vi "STED Control V15.vi"() -> ()   [LabVIEW 2014]
uses:
  Controls/Button 2.ctl
  Type Defs/Image Acquisition Parameters.ctl
  Laser Controls.ctl
  Detectors.ctl
  Type Defs/P541.ctl
  Type Defs/M227.ctl
  Type Defs/P612.ctl
  Type Defs/M686.ctl
  Type Defs/P841.ctl
  Type Defs/ASI.ctl
  Type Defs/N664_V2.ctl
  Type Defs/STED Graph Controls.ctl
  Type Defs/Display Controls.ctl
  Type Defs/Z comp.ctl
  FPGA-7842R-Reference.ctl
  Manual Controls V2.ctl
  Scan Parameters.ctl
  <vilib>/Utility/miscctls.llb/LVPositionTypeDef.ctl
  Controls/StageStates.ctl
  DM_Dual_V2/Controls/Standard Action.ctl
  Focus Lock/Controls/Counter Action.ctl
  Focus Lock/Controls/Standard Action for Focus Lock.ctl
  <vilib>/Utility/miscctls.llb/LVRectTypeDef.ctl
  <vilib>/event_ctls.llb/lveventtype.ctl
  <vilib>/Utility/file.llb/Read From Spreadsheet File (DBL).vi
  <vilib>/FPGAPlugInAG/PCIe-7841R/niLvFpga_Open_PCIe-7841R.vi
  <vilib>/FPGAPlugInAG/PCIe-7841R/niLvFpga_Close_PCIe-7841R.vi
  <vilib>/Utility/file.llb/Write To Spreadsheet File (DBL).vi
  <vilib>/rvi/interface/nirviOpenFPGA/nirviOpenFPGA.xnode
  FPGA Bitfiles/MainSTEDFPGAProj_FPGATarget_WaveformandLaser_VYICzb2jDIA.lvbitx
  FPGA Target VIs/FPGA-7841R/Waveform and Laser Controls V6.vi
  <vilib>/rvi/interface/nirviCloseFPGA/nirviCloseFPGA.xnode
panel:
  in  "Wake Up FPGA":bool
  in  "z Comp.":T1
  out "Graph Ref Out":refnum<vi>[](array[refnum])
  out "Frame Counter":i32
  in  "Follow Cursor":bool
  in  "Laser Controls 2":T2={"Laser On Time (Ticks)"=16, "Laser Delay (Ticks)"=3}
  out "Channel 6":sgl[][](graph)
  out "Channel 5":sgl[][](graph)
  out "Channel 4":sgl[][](graph)
  out "Channel 3":sgl[][](graph)
  out "Channel 2":sgl[][](graph)
  out "Channel 1":sgl[][](graph)
  in  "Display Controls":T3
  in  "Graph Tools":T4={"Zoom Out"=FALSE, "Zoom In"=FALSE, "Reset Zoom"=FALSE, "Pan Tool"=FALSE, "Show Cursor"=FALSE, "Load File"=FALSE, "Fit Tool"=FALSE, "Smooth Tool"=FALSE, "Merge Tool"=FALSE, "Auto Scale"=FALSE, "Apply Color"=FALSE, "Color Map"=enum."Fire"}
  in  "Shutters":T5
  in  "Upper Objective Z - N664":T6={"Up N664"=FALSE, "Down N664"=FALSE, "Step Size (um)"=0.001, "Position (mm)"=0.0, "Home"=FALSE, "Save"=FALSE} {"Step Size (um)" min=0.001}
  in  "Cavity Translation Z - ASI":T7={"Up ASI"=FALSE, "Down ASI"=FALSE, "Step Size (um)"=0.001, "Z (um)"=0.001, "F (um)"=0.001, "Velocity"=0.001} caption="ASI" {"Velocity" min=0.001; "F (um)" min=0.001; "Z (um)" min=-1500.0 max=1500.0; "Step Size (um)" min=0.001}
  in  "Phase Comp Mirror - P841":T8={"Position (µm)"=0.0, "Step Size (µm)"=0.05, "Up P841"=FALSE, "Down P841"=FALSE}
  in  "Sample Stage XY - M686":T9={"Home Button"=FALSE, "Left Button"=FALSE, "Down Button"=FALSE, "Right Button"=FALSE, "Up Button"=FALSE, "X"=0.0, "Y"=0.0, "Step Size (um)"=1.0} {"Y" format="%#_8g"; "X" format="%#_8g"}
  in  "Bottom Objective XY - P612":T10
  in  "Abort AllStage":bool
  in  "Stages":T11={"M227"=TRUE, "N664"=TRUE, "P612"=TRUE, "M686"=TRUE, "P841"=TRUE, "ASI"=FALSE}
  in  "Sample Z Coarse - M227":T12
  in  "Tab Control":T13(tab)
  in  "SLM":T14
  in  "DM":T14
  in  "Timing":T14
  in  "Focus Lock":T14
  in  "Sequence":T14
  in  "Stage Monitor":T14
  in  "Camera":T14
  in  "Sequence Cluster":T15
  in  "Sample Z - P541":T16={"Step Up"=FALSE, "Step Down"=FALSE, "Z Position"=0.0, "Step Size (um)"=1.0, "Home"=FALSE, "Save"=FALSE}
  in  "Detectors":T17={"PMT"=TRUE, "Far Red (685/40 nm)"=FALSE, "Orange (624/40 nm)"=FALSE, "Green (525/50 nm)"=FALSE, "Sum All"=FALSE}
  in  "Laser Controls":T18 {"STED Power (V)" scale=0.0..10.0}
  in  "Save File Path":path=path "C:/isoSTED_Data/Temp/Test_0000.dbl"
  in  "Capture":bool
  in  "Image Acquisition Parameters":T19={"Scan Type"=enum."Beam Scanning", "Scan Mode"=enum."XY", "Fast Axis Frequency (Hz)"=15780.0, "Image Format"=256, "Line Accumulations"=100, "Frames Per Capture"=1, "Frames Accumulations"=1, "Image Dimension (um)"=[15.0, 15.0], "Number of Z Steps"=1, "Z Steps Size (um)"=1.0, "Pixel Size (nm)"=[58.59375, 58.59375], "Customized Image Format"=[]} {"Z Steps Size (um)" min=0.0; "Number of Z Steps" min=1; "Frames Accumulations" min=1; "Frames Per Capture" min=1; "Line Accumulations" min=1; "Image Format" items=["64 x 64"=64, "128 x 128"=128, "256 x 256"=256, "512 x 512"=512, "1024 x 1024"=1024, "2048 x 2048"=2048, "Customized..."=0]}
  in  "Live":T14
  in  "Exit":bool
  # "Piston"
  # "Defocus"
  # "Spherical"
  # "Frame Mode"
  # "Line Mode"
  # "Length"
  # "Height"
  # "XY"
  # "Z"
  # "Length"
  # "Height"
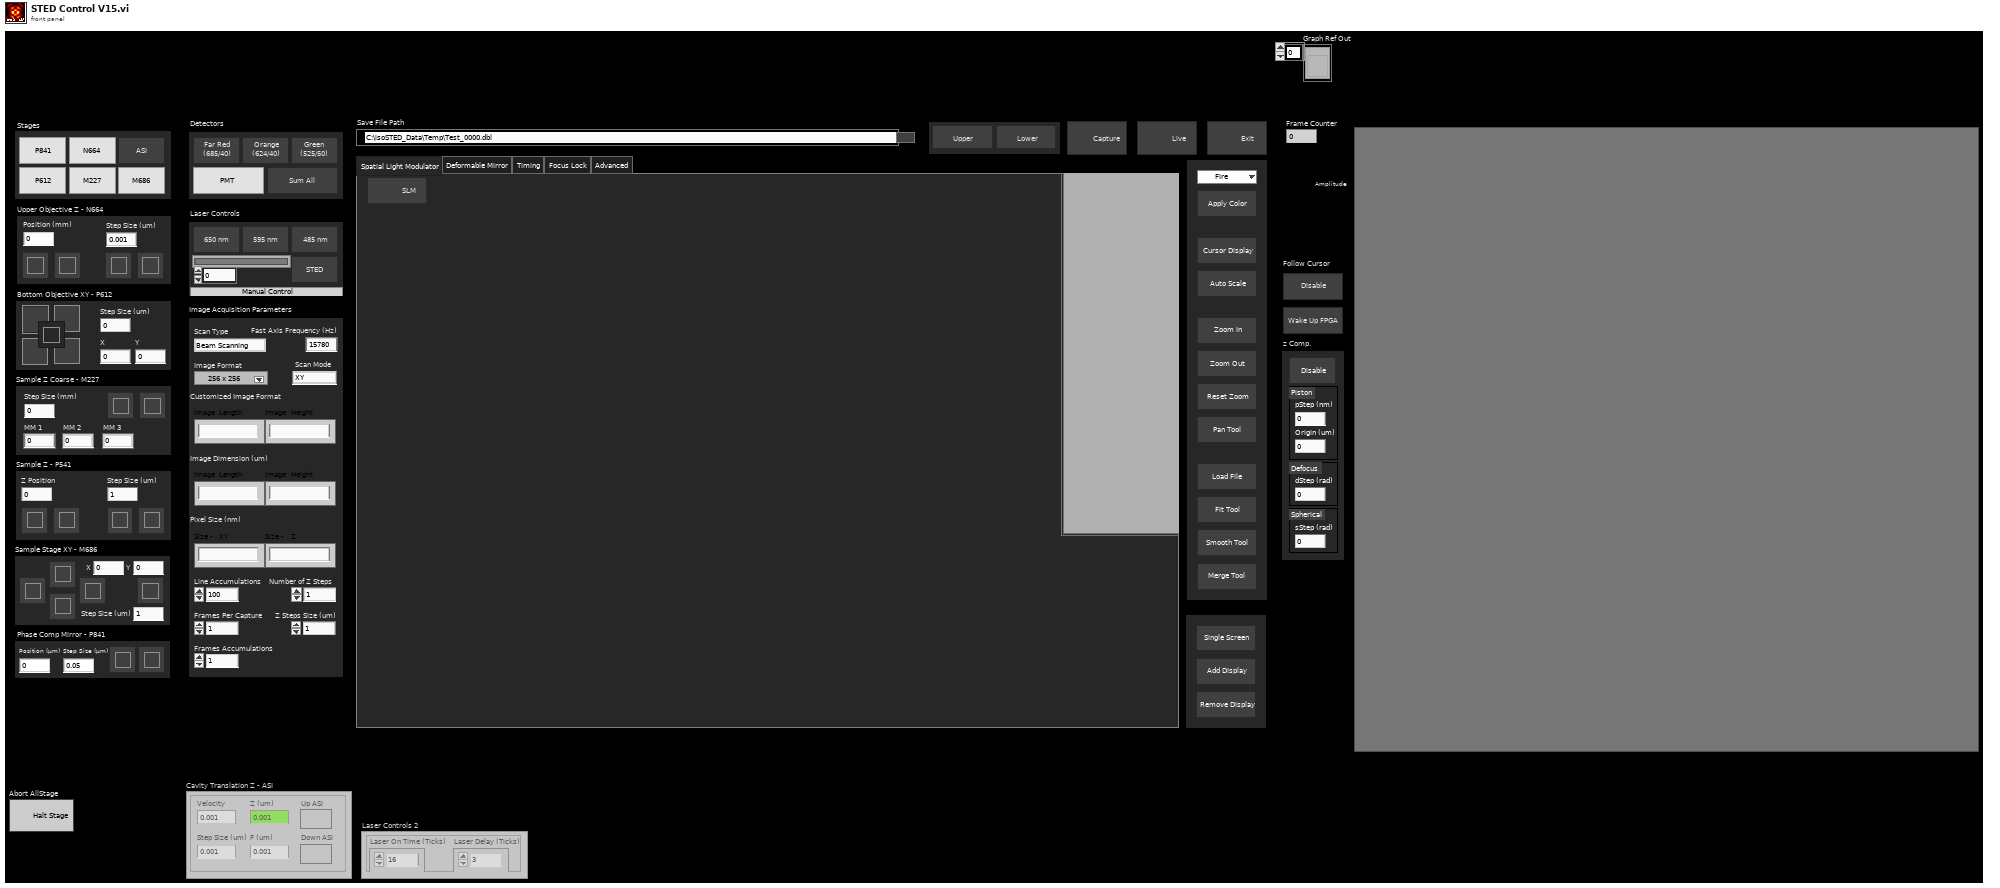
[diagram p1: front panel]
types:
  T1 = typedef "Z comp.ctl" = cluster{"Enable":bool, "pStep (nm)":dbl, "Origin (um)":dbl, "dStep (rad)":dbl, "sStep (rad)":dbl}
  T2 = cluster{"Laser On Time (Ticks)":i8, "Laser Delay (Ticks)":i8}
  T3 = typedef "Display Controls.ctl" = cluster{"Remove Display":bool, "Add Display":bool, "Single Screen":bool}
  T4 = typedef "STED Graph Controls.ctl" = cluster{"Zoom Out":bool, "Zoom In":bool, "Reset Zoom":bool, "Pan Tool":bool, "Show Cursor":bool, "Load File":bool, "Fit Tool":bool, "Smooth Tool":bool, "Merge Tool":bool, "Auto Scale":bool, "Apply Color":bool, "Color Map":enum16{"System", "Fire", "Gray", "Red", "Green", "Blue", "Cyan", "Magenta", "Yellow", "Red-White", "Green-White", "Blue-White", "Glow"}}
  T5 = cluster{"Upper Shutter":bool, "Lower Shutter":bool}
  T6 = typedef "N664_V2.ctl" = cluster{"Up N664":bool, "Down N664":bool, "Step Size (um)":dbl, "Position (mm)":dbl, "Home":bool, "Save":bool}
  T7 = typedef "ASI.ctl" = cluster{"Up ASI":bool, "Down ASI":bool, "Step Size (um)":dbl, "Z (um)":dbl, "F (um)":dbl, "Velocity":dbl}
  T8 = typedef "P841.ctl" = cluster{"Position (µm)":dbl, "Step Size (µm)":dbl, "Up P841":bool, "Down P841":bool}
  T9 = typedef "M686.ctl" = cluster{"Home Button":bool, "Left Button":bool, "Down Button":bool, "Right Button":bool, "Up Button":bool, "X":dbl, "Y":dbl, "Step Size (um)":dbl}
  T10 = typedef "P612.ctl" = cluster{"Home Button":bool, "Up Button":bool, "Left Button":bool, "Down Button":bool, "Right Button":bool, "Step Size (um)":dbl, "X":dbl, "Y":dbl}
  T11 = cluster{"M227":bool, "N664":bool, "P612":bool, "M686":bool, "P841":bool, "ASI":bool}
  T12 = typedef "M227.ctl" = cluster{"Up M227":bool, "Down M227":bool, "Step Size (mm)":dbl, "MM 1":dbl, "MM 2":dbl, "MM 3":dbl}
  T13 = enum32{"Spatial Light Modulator", "Deformable Mirror", "Timing", "Focus Lock", "Advanced"}
  T14 = typedef "Button 2.ctl" = bool
  T15 = cluster{"Operation Option":enum32{"frameSeq", "lineSeq"}, "AddSeq":bool, "DeleteSeq":bool, "DeleteAllSeq":bool, "Sequence List":enum32{"Seq 1", "Seq 2", "Seq 3", "Seq 4"}}
  T16 = typedef "P541.ctl" = cluster{"Step Up":bool, "Step Down":bool, "Z Position":dbl, "Step Size (um)":dbl, "Home":bool, "Save":bool}
  T17 = typedef "Detectors.ctl" = cluster{"PMT":bool, "Far Red (685/40 nm)":bool, "Orange (624/40 nm)":bool, "Green (525/50 nm)":bool, "Sum All":bool}
  T18 = typedef "Laser Controls.ctl" = cluster{"STED Power (V)":dbl, "STED":bool, "650 nm":bool, "590 nm":bool, "485 nm":bool, "Manual Control":bool}
  T19 = typedef "Image Acquisition Parameters.ctl" = cluster{"Scan Type":enum16{"Sample Scanning", "Beam Scanning"}, "Scan Mode":enum16{"XY", "XZ", "YZ", "XYZ"}, "Fast Axis Frequency (Hz)":dbl, "Image Format":u16, "Line Accumulations":u16, "Frames Per Capture":u16, "Frames Accumulations":u16, "Image Dimension (um)":dbl[], "Number of Z Steps":u8, "Z Steps Size (um)":dbl, "Pixel Size (nm)":dbl[], "Customized Image Format":dbl[]}
  T20 = typedef "Scan Parameters.ctl" = cluster{"Fast_Ax_Amp_V":dbl, "Fast_Ax_Off_V":dbl, "Slow_Ax_Amp_V":dbl, "Slow_Ax_Off_V ":dbl, "Slow_Ax_Max_V_VperS":dbl, "Slow_Ax1_Del25ns":i32, "Slow_Ax2_Del25ns":i32, "Stage_X_Off_V":dbl, "Stage_Y_Off_V":dbl, "Stage_Z_Off_V":dbl, "Galvo1_Off_V":dbl, "Galvo2_Off_V":dbl, "Last_Scan_Mode":enum16{"XY", "XZ", "YZ", "XYZ"}, "Current_Scan_Mode":enum16{"XY", "XZ", "YZ", "XYZ"}, "Fly_Back_Lines":u16, "Linear_Ramp_End":u32, "Z_Step_I16":i16, "Z_Start_I16":i16, "Laser_States _U32":u32, "590_Voltage_I16":i16, "775_AOM_Volt_I16":i16, "Blanking OFF":bool, "Unused_Axis_I16":i16}
  T21 = typedef "Manual Controls V2.ctl" = cluster{"Galvo 1 Position (I16)":i16, "Galvo 2 Position (I16)":i16, "X Axis Voltage (I16)":i16, "Y Axis Voltage (I16)":i16, "Z Axis Voltage (I16)":i16, "Res Mirror Amp (I16)":i16, "Res Mirror Mute":bool, "Upper Shutter":bool, "Lower Shutter":bool}
  T22 = typedef "FPGA-7842R-Reference.ctl" = enum16{"Stage Control", "Laser Control", "Unused Axis I16", "Exit", "Set Res Mirror", "Set Galvo", "Current Frame for Capture", "Default", "Close FPGA", "Stop Waveforms", "Start Waveforms", "Shutter Control", "Initialize"}
  T23 = typedef "Counter Action.ctl" = enum16{"Zero", "Plus One", "Read"}
  T24 = typedef "StageStates.ctl" = enum16{"POSITION", "MVR", "MOVE", "HALT", "ONTARGET", "ERROR", "EXIT", "HOME", "ZEROPOS", "NANOPOS", "QUIT", "ANALOG"}
  T25 = enum8{"Enabled", "Disabled", "Disabled and Grayed Out"}
  T26 = typedef "Standard Action.ctl" = enum16{"Read", "Write"}
  T27 = typedef "Standard Action for Focus Lock.ctl" = enum16{"Read", "Write"}
  T28 = typedef "LVRectTypeDef.ctl" = cluster{"Left":i16, "Top":i16, "Right":i16, "Bottom":i16}
  T29 = enum32{"Invalid", "Standard", "Closed", "Hidden", "Minimized", "Maximized"}
  T30 = typedef "lveventtype.ctl" = enum32{"Null", "Timeout", "Annotation Menu Selection", "Annotation Menu Selection?", "App Instance Close", "App Instance Close?", "Autoscale Range Change", "Bookmark Info Change", "Cell Edit", "Cell Edit?", "Cursor Grab", "Cursor Grab?", "Cursor Menu Selection", "Cursor Menu Selection?", "Cursor Move", "Cursor Release", "Data Change", "Direction Change", "Display State Change", "Drag Ended", "Drag Enter", "Drag Leave", "Drag Over", "Drag Source Update", "Drag Starting", "Drag Starting?", "Drop", "Exec State Change", "Key Down", "Key Down?", "Key Repeat", "Key Repeat?", "Key Up", "Listbox Double Click", "Menu Activation?", "Menu Selection (App)", "Menu Selection? (App)", "Menu Selection (User)", "Mouse Down", "Mouse Down?", "Mouse Enter", "Mouse Leave", "Mouse Move", "Mouse Up", "Mouse Wheel", "NI Security User Change (App)", "Pane Size", "Panel Close", "Panel Close?", "Panel Resize", "Plot Attribute Change", "Scale Range Change", "Shortcut Menu Activation?", "Shortcut Menu Selection (App)", "Shortcut Menu Selection? (App)", "Shortcut Menu Selection (User)", "Tree Double Click", "Tree Drag", "Tree Drag?", "Tree Drop", "Tree Drop?", "Tree Item Close", "Tree Item Close?", "Tree Item Open", "Tree Item Open?", "User Event", "Value Change"}
  T31 = typedef "LVPositionTypeDef.ctl" = cluster{"Left":i32, "Top":i32}
  T32 = cluster{"Upper Shutter":bool, "Upper Shutter":bool}
  T33 = cluster{bool, bool, dbl, "Numeric":dbl, "Numeric":dbl, "Numeric":dbl}
  T34 = cluster{"Down_N664":bool, "Down_N664":bool, "Step Size (um)":dbl, "Numeric":dbl, bool, bool}
  T35 = cluster{bool, bool, bool, bool, bool, dbl, "Numeric":dbl, "Numeric":dbl}
  T36 = cluster{bool, bool, bool, bool, bool, "Numeric":dbl, "Numeric":dbl, dbl}
  T37 = cluster{"Enable":bool, "pStep (nm)":bool, "Origin (um)":bool, "dStep (rad)":bool, "sStep (rad)":bool}
  T38 = typedef "MirrorModes_DUAL.ctl" = cluster{"Mode":string, "Amplitude":dbl}[][]
  T39 = cluster{"Detectors Parameters Out":T17, "Laser Parameters Out":T18, "Image Acquisition Parameters Out":T19}[]
  T40 = cluster{"Detectors Parameters Out":T17, "Laser Parameters Out":T18, "Image Acquisition Parameters Out":T19}
  T41 = cluster{"Scan Type":bool, "Scan Mode":bool, "Fast Axis Frequency (Hz)":bool, "Image Format":bool, "Line Accumulations":bool, "Frames Per Capture":bool, "Frames Accumulations":bool, "Image Dimension (um)":bool[], "Number of Z Steps":bool, "Z Steps Size (um)":bool, "Pixel Size (nm)":bool[], "Customized Image Format":bool[]}
  T42 = typedef "Focus Lock.ctl" = cluster{"EXIT":bool, "Lock Current":bool, "Manual":bool, "Drift":bool, "Move":bool, "Control Option":bool}
  T43 = typedef "LVAllMonitorsDisplayTypeDef.ctl" = cluster{"Bounds":cluster{"Left":i16, "Top":i16, "Right":i16, "Bottom":i16}, "Depth":i16}[]
  T44 = cluster{"Bounds":cluster{"Left":i16, "Top":i16, "Right":i16, "Bottom":i16}, "Depth":i16}
  T45 = enum16{"System", "Fire", "Gray", "Red", "Green", "Blue", "Cyan", "Magenta", "Yellow", "Red-White", "Green-White", "Blue-White", "Glow"}
  T46 = typedef "LVPointDoubleTypeDef.ctl" = cluster{"Cursor X":dbl, "Cursor Y":dbl}
  T47 = typedef "LVRangeTypeDef.ctl" = cluster{"Minimum":dbl, "Maximum":dbl, "Increment":dbl, "Minor Increment":dbl, "Start":dbl}
  T48 = cluster{"Operation Option":bool, "AddSeq":bool, "DeleteSeq":bool, "DeleteAllSeq":bool, "Sequence List":bool}
  T49 = typedef "IMAQ Image.ctl" = refnum<image>
  T50 = typedef "Waveform Data.ctl" = cluster{"Waveform Scan Parameters":cluster{"Scanning Mode":u8, "Fast Axis WF Length (Elements)":i32, "Fast Axis Sample Period (Ticks)":u32, "Slow Axis 1 WF Length (Elements)":i32, "Slow Axis 1 Sample Period (Ticks)":u32, "Slow Axis 1 Delay (25 ns) Steps":i32, "Slow Axis 2 WFLength (Elements)":i32, "Slow Axis 2 Sample Period (Ticks)":u32, "Slow Axis 2 Delay (25 ns) Steps":i32}, "Fast Axis Waveform":dbl[], "Slow Axis 1 Waveform":dbl[], "Slow Axis 2 Waveform":dbl[]}
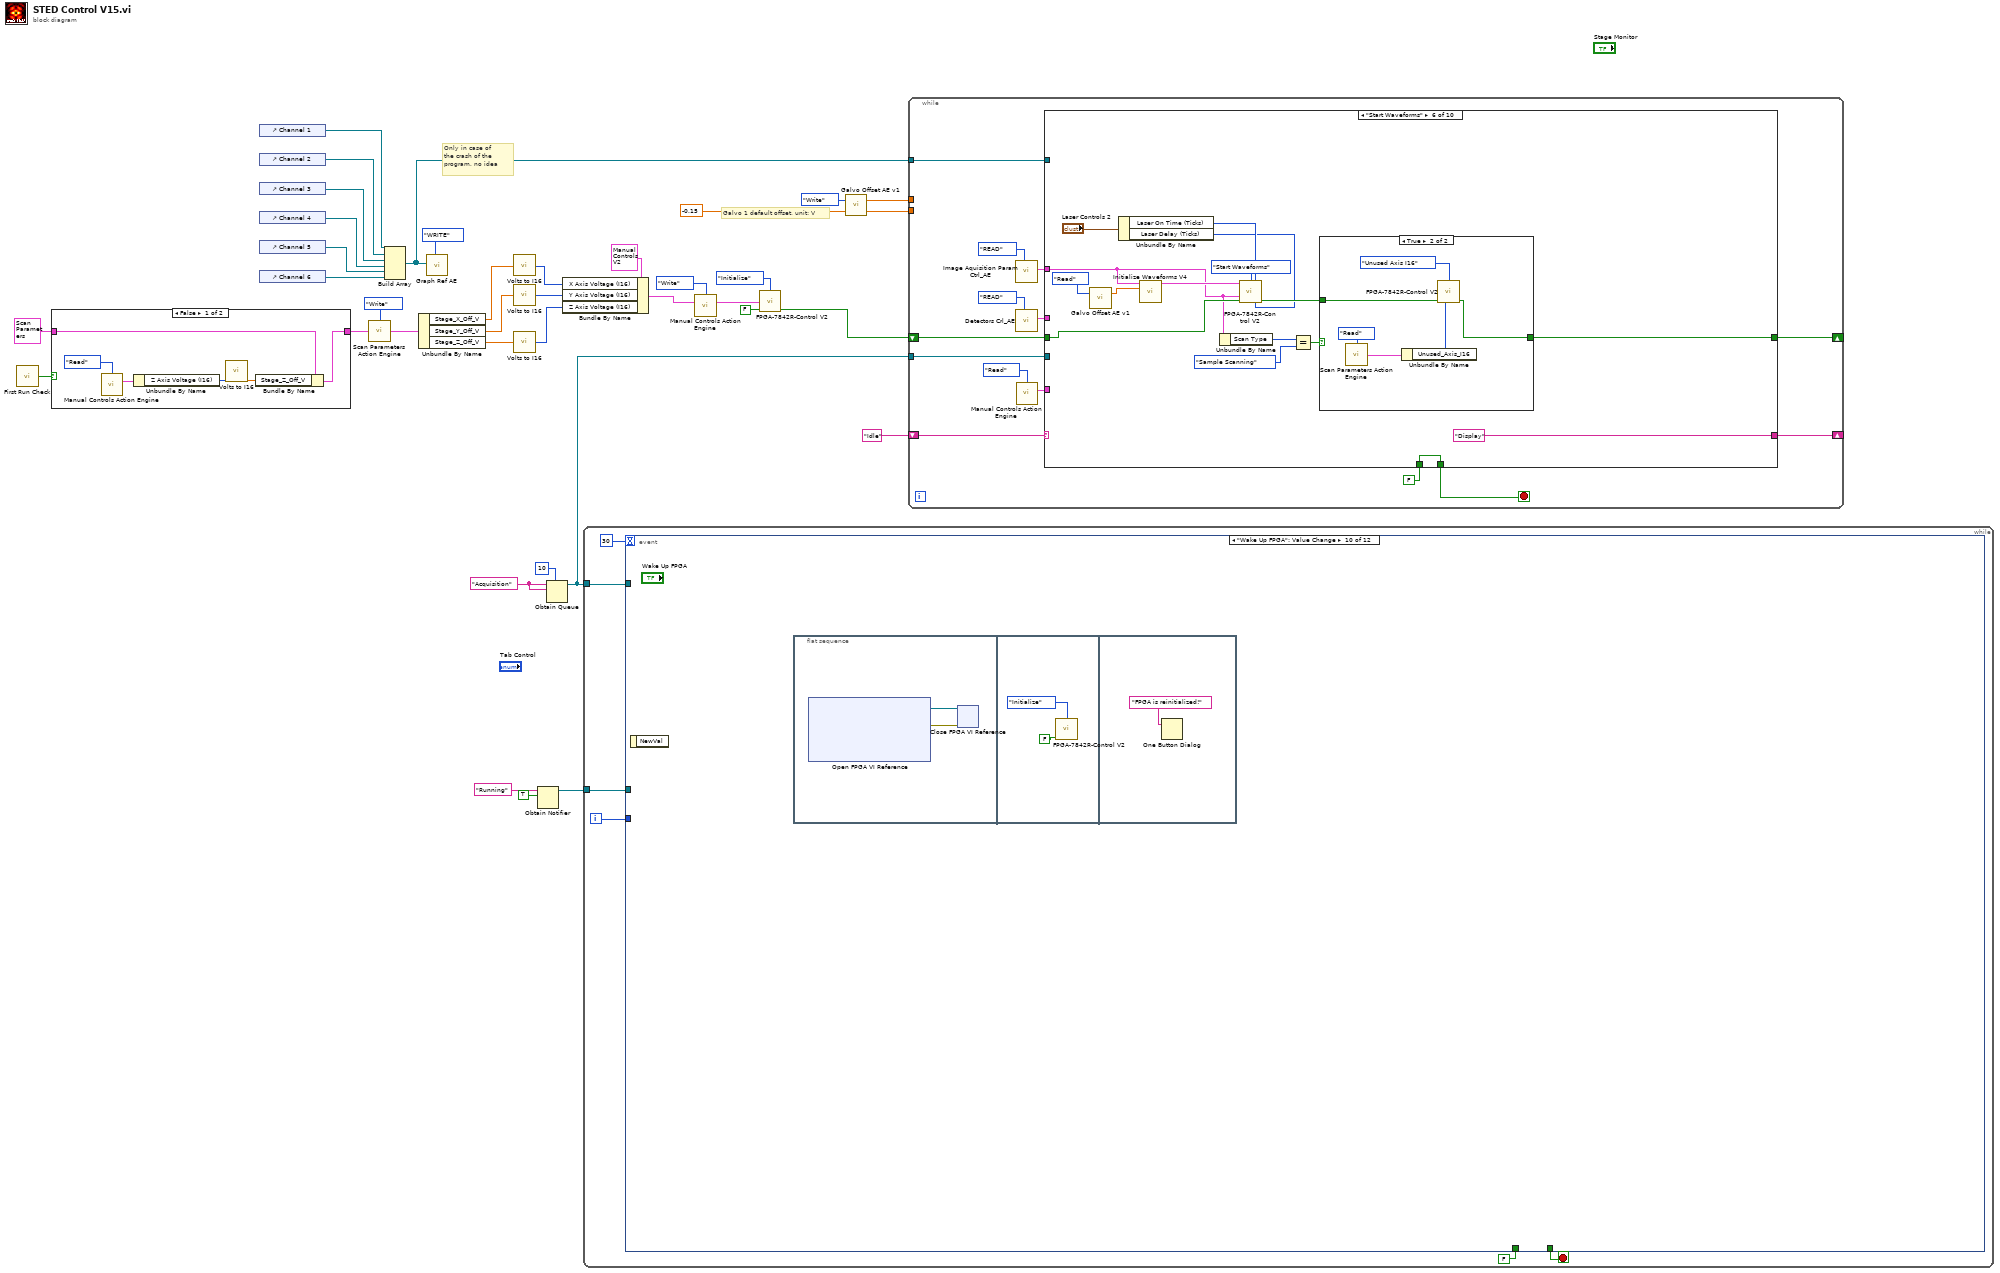
[diagram p0: block diagram]
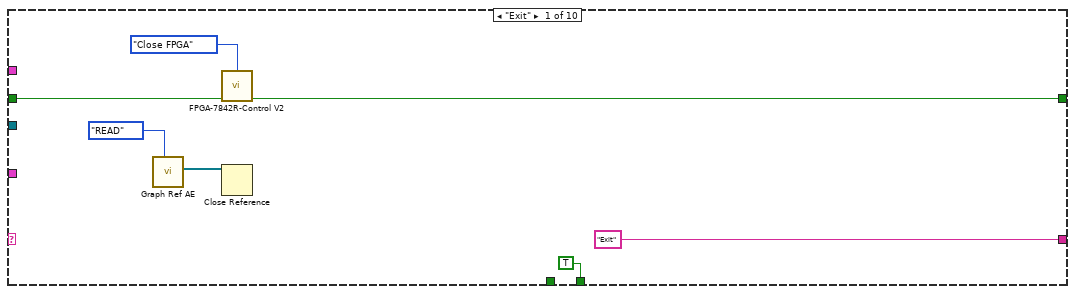
[diagram p3: hidden frame]
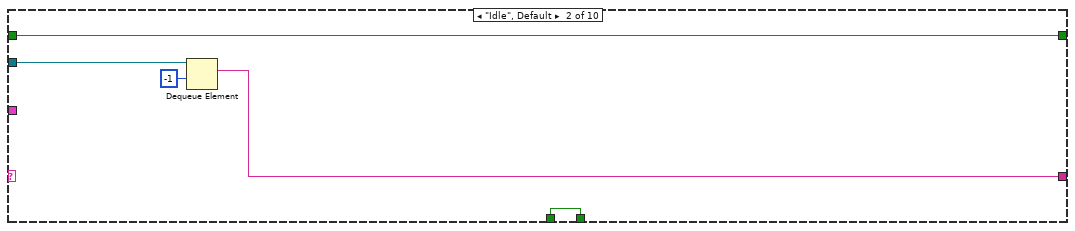
[diagram p4: hidden frame]
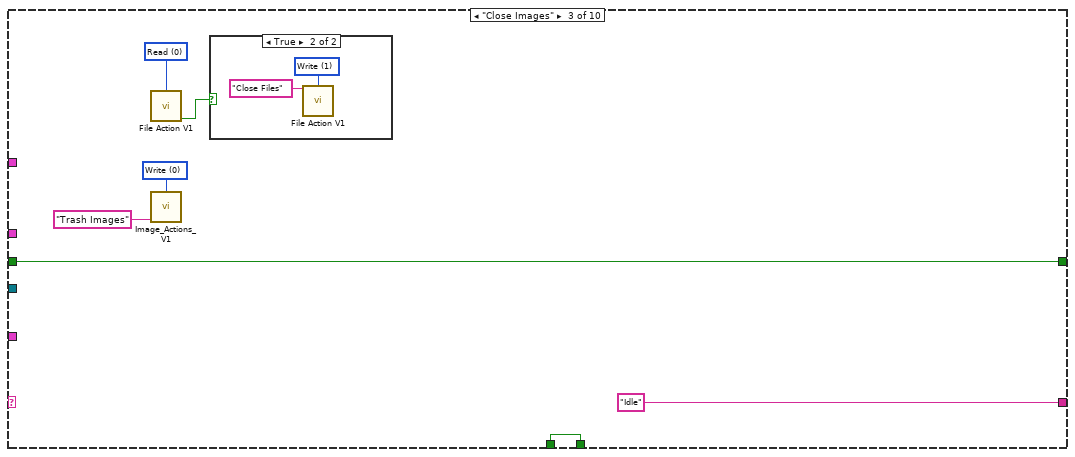
[diagram p5: hidden frame]
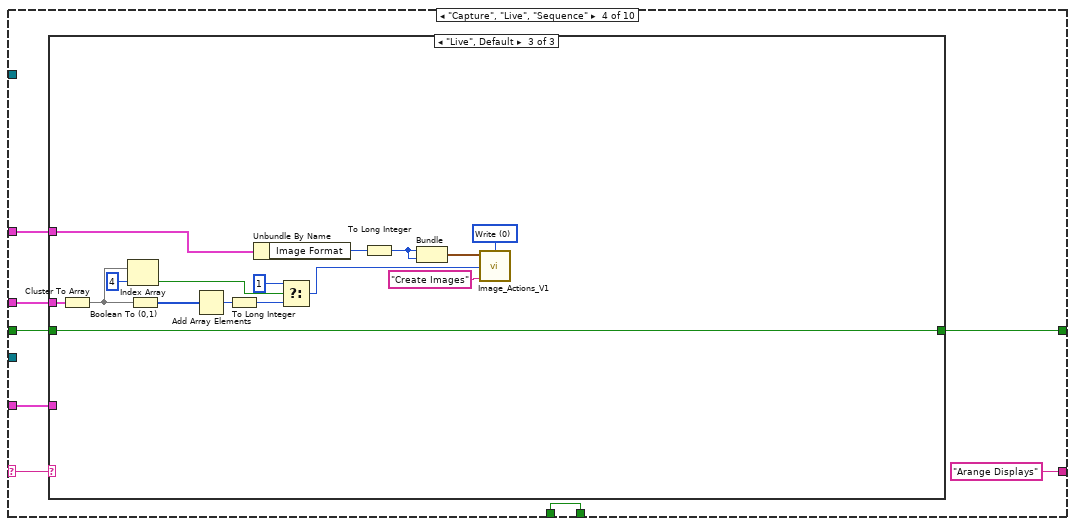
[diagram p7: hidden frame]
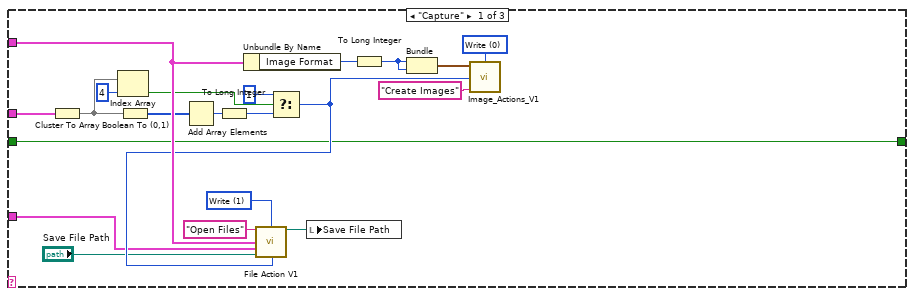
[diagram p8: hidden frame]
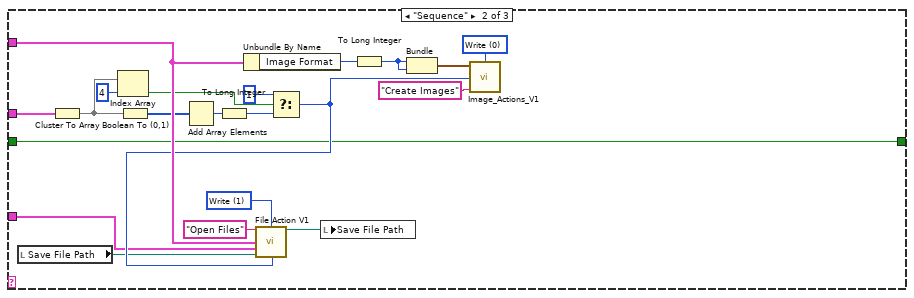
[diagram p9: hidden frame]
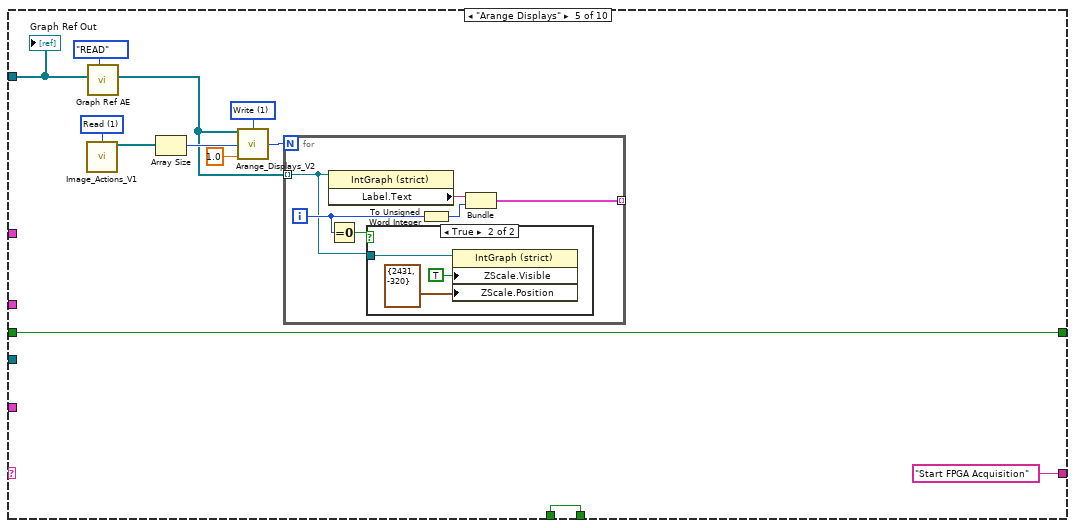
[diagram p10: hidden frame]
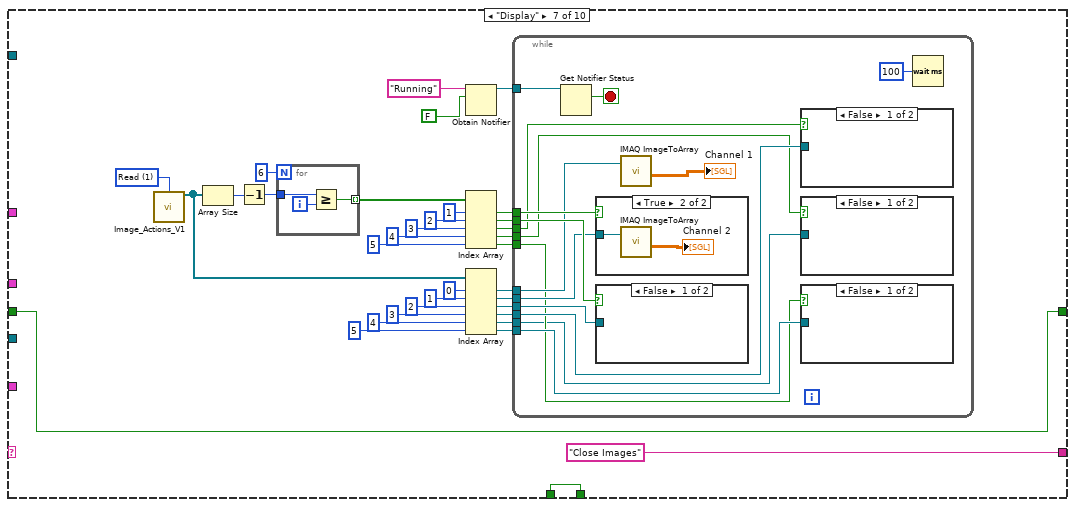
[diagram p13: hidden frame]
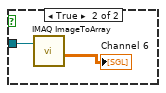
[diagram p14: hidden frame]
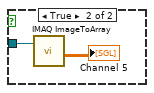
[diagram p15: hidden frame]
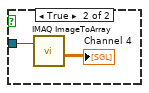
[diagram p16: hidden frame]
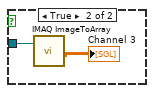
[diagram p17: hidden frame]
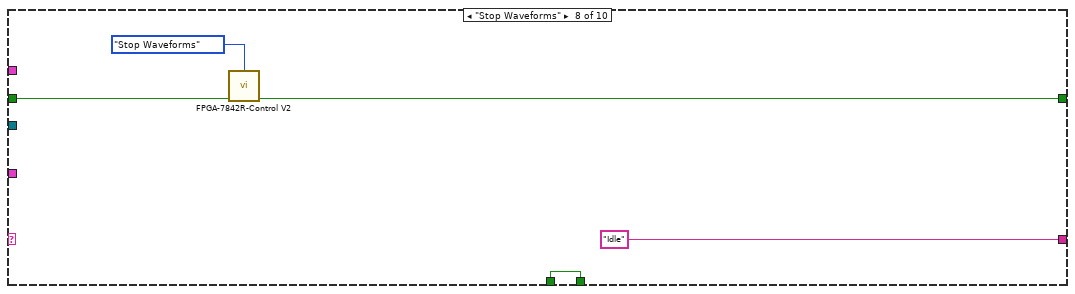
[diagram p19: hidden frame]
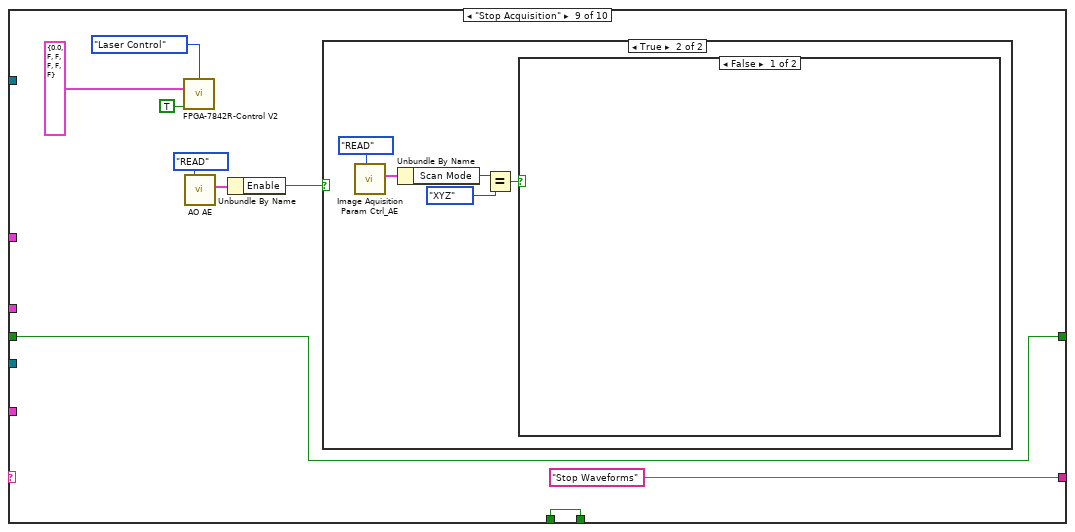
[diagram p20: hidden frame]
diagram:
  w20 = "Acquisition" ("name (unnamed)")
  # "Galvo 1 default offset, unit: V"
  # "Only in case of \nthe crash of the\nprogram, no idea"
  n1 = call "First Run Check.vi"() -> ("First Run?"=w14:bool)  [unwired: 15 in]
  n2 = case shown="False" w14 {
    tunnel: T20 {"Fast_Ax_Amp_V"=0.0, "Fast_Ax_Off_V"=0.0, "Slow_Ax_Amp_V"=0.0, "Slow_Ax_Off_V "=0.0, "Slow_Ax_Max_V_VperS"=0.0, "Slow_Ax1_Del25ns"=0, "Slow_Ax2_Del25ns"=0, "Stage_X_Off_V"=5.0, "Stage_Y_Off_V"=5.0, "Stage_Z_Off_V"=5.0, "Galvo1_Off_V"=0.0, "Galvo2_Off_V"=0.0, "Last_Scan_Mode"=enum."XY", "Current_Scan_Mode"=enum."XY", "Fly_Back_Lines"=0, "Linear_Ramp_End"=0, "Z_Step_I16"=0, "Z_Start_I16"=0, "Laser_States _U32"=0, "590_Voltage_I16"=0, "775_AOM_Volt_I16"=0, "Blanking OFF"=FALSE, "Unused_Axis_I16"=16384} ("Scan Parameters IN") -> [w43 w44]
    tunnel: [w38 w44] -> w12
    frame False {
      n3 = call "Manual Controls Action Engine.vi"("Action"=enum16{"Read", "Write"}."Read") -> ("Manual Controls Out"=w41:T21)  [unwired: 14 in]
      n4 = Unbundle By Name(w41) -> ("Z Axis Voltage (I16)"=w42:i16)
      n5 = call "Volts to I16.vi"("Volatge (I16)"=w42) -> ("Voltage (V)"=w39:dbl)  [unwired: 13 in, 1 out]
      n6 = Bundle By Name(cluster=w43, "Stage_Z_Off_V"=w39) -> (w38:T20)
    }
    frame True {
    }
  }
  n7 = control-ref of="Channel 1"() -> (w9:refnum<vi>)
  n8 = control-ref of="Channel 2"() -> (w10:refnum<vi>)
  n9 = control-ref of="Channel 3"() -> (w11:refnum<vi>)
  n10 = control-ref of="Channel 4"() -> (w6:refnum<vi>)
  n11 = control-ref of="Channel 5"() -> (w8:refnum<vi>)
  n12 = control-ref of="Channel 6"() -> (w7:refnum<vi>)
  n13 = call "Scan Parameters Action Engine.vi"("Action"=enum16{"Read", "Write"}."Write", "Scan Parameters IN"=w12) -> ("Scan Parameters OUT"=w30:T20)  [unwired: 13 in]
  n14 = Build Array(w9, w10, w11, w6, w8, w7) -> (w5:refnum<vi>[])
  n15 = Unbundle By Name(w30) -> ("Stage_X_Off_V"=w26:dbl, "Stage_Y_Off_V"=w25:dbl, "Stage_Z_Off_V"=w24:dbl)
  n16 = call "Graph Ref AE.vi"("Action"=enum16{"READ", "WRITE"}."WRITE", "Graph Ref In"=w5) -> ()  [unwired: 9 in, 1 out]
  n17 = call "Volts to I16.vi"("Voltage (V)"=w26) -> ("I16"=w27:i16)  [unwired: 13 in, 1 out]
  n18 = call "Volts to I16.vi"("Voltage (V)"=w25) -> ("I16"=w28:i16)  [unwired: 13 in, 1 out]
  n19 = call "Volts to I16.vi"("Voltage (V)"=w24) -> ("I16"=w29:i16)  [unwired: 13 in, 1 out]
  n20 = Obtain Notifier(name (unnamed)="Running", notification data type=TRUE) -> (notifier out=w16:refnum<notifier>)  [unwired: 2 in, 2 out]
  n21 = Obtain Queue(max queue size (-1, unlimited)=10, name (unnamed)=w20, element data type=w20) -> (queue out=w22:refnum<queue>)  [unwired: 2 in, 2 out]
  n22 = Bundle By Name(cluster=T21 {"Galvo 1 Position (I16)"=-280, "Galvo 2 Position (I16)"=0, "X Axis Voltage (I16)"=16384, "Y Axis Voltage (I16)"=16384, "Z Axis Voltage (I16)"=16384, "Res Mirror Amp (I16)"=0, "Res Mirror Mute"=FALSE, "Upper Shutter"=FALSE, "Lower Shutter"=FALSE} ("Manual Controls"), "X Axis Voltage (I16)"=w27, "Y Axis Voltage (I16)"=w28, "Z Axis Voltage (I16)"=w29) -> (w31:T21)
  n23 = while {
    tunnel: w22 -> [w48]
    tunnel: w16 -> [w45]
    i -> [w46]
    stop <- w50 stop-if-true
    n24 = event shown="[9] \"Wake Up FPGA\": Value Change" {
      selector: _ -> [_ _ _ _ _ _ _ _ _ _ _ _]
      dyn-events: _ -> [_ _ _ _ _ _ _ _ _ _ _ _]
      timeout: 30 -> [_ _ _ _ _ _ _ _ _ _ _ _]
      tunnel: [w58 _ w265 w335 w500 _ w848 w947 w1162 _ _ w1293] -> w50
      tunnel: FALSE -> [w58 _ w265 w335 w500 _ w848 w947 w1162 _ _ _]
      tunnel: w48 -> [w55 _ w264 _ _ _ _ _ _ _ _ w1292]
      tunnel: w46 -> [w53 _ _ _ _ _ _ _ _ _ _ _]
      tunnel: w45 -> [w51 _ w262 _ _ _ _ _ _ _ _ w1286]
      event Timeout {
        n25 = event-data() -> ()  [unwired: 1 in, 3 out]
        n26 = Equal To 0?(x=w53) -> (x = 0?=w52:bool)
        n27 = Get Notifier Status(notifier=w51) -> (current notification=w57:bool)  [unwired: 1 in, 4 out]
        n28 = case shown="True" w52 {
          frame False {
            w68 = enum16{"WRITE", "READ", "HOME", "SAVE HOME"}."READ" ("Enum")
            n29 = call "AO AE.vi"("Action"=enum16{"READ", "WRITE"}."READ") -> ("Z Comp. Output"=w61:T1)  [unwired: 8 in, 2 out]
            n30 = Unbundle By Name(w61) -> ("Enable"=w66:bool, "Origin (um)"=w62:dbl, "pStep (nm)"=w63:dbl, "dStep (rad)"=w60:dbl, "sStep (rad)"=w59:dbl)
            n31 = call "Image Aquisition Param Ctrl_AE.vi"("Action"=enum16{"READ", "WRITE"}."READ") -> ("Image Acquisition Parameters Out"=w102:T19)  [unwired: 10 in]
            n32 = call "Detectors Crl_AE.vi"("Action"=enum16{"READ", "WRITE"}."READ") -> ("Detectors Parameters Out"=w103:T17)  [unwired: 10 in]
            n33 = call "LASERs_ Crl_AE.vi"("Action"=enum16{"READ", "WRITE"}."READ") -> ("Laser Parameters Out"=w104:T18)  [unwired: 10 in]
            n34 = local write "z Comp."(w61) -> ()
            n35 = local write "Image Acquisition Parameters"(w102) -> ()
            n36 = local write "Detectors"(w103) -> ()
            n37 = local write "Laser Controls"(w104) -> ()
            n38 = call "Frame Counter.vi"("Action"=Counter_Action."Read") -> ("Num"=w67:i32)
            "Frame Counter" <- w67
            n39 = case shown="False" w66 {
              tunnel: w67 -> [_ w108]
              tunnel: w63 -> [_ w109]
              tunnel: w62 -> [_ w107]
              tunnel: w61 -> [_ _]
              tunnel: w60 -> [_ w106]
              tunnel: w59 -> [_ w105]
              frame False {
              }
              frame True {
                n40 = local read "Capture"() -> (w116:bool)
                n41 = local read "Live"() -> (w117:T14)
                n42 = call "Image Aquisition Param Ctrl_AE.vi"("Action"=enum16{"READ", "WRITE"}."READ") -> ("Image Acquisition Parameters Out"=w118:T19)  [unwired: 10 in]
                n43 = Or(x=w116, y=w117) -> (x .or. y?=w113:T14)
                n44 = Unbundle By Name(w118) -> ("Scan Mode"=w115:enum16{"XY", "XZ", "YZ", "XYZ"}, "Number of Z Steps"=w110:u8)
                n45 = Equal?(x=enum16{"XY", "XZ", "YZ", "XYZ"}."XYZ", y=w115) -> (x = y?=w112:bool)
                n46 = And(x=w113, y=w112) -> (x .and. y?=w111:T14)
                n47 = case shown="True" w111 {
                  tunnel: w108 -> [_ w129]
                  tunnel: w110 -> [_ w128]
                  tunnel: w109 -> [_ w127]
                  tunnel: w107 -> [_ w126]
                  tunnel: w106 -> [_ w121]
                  tunnel: w105 -> [_ w120]
                  frame False {
                  }
                  frame True {
                    n48 = Quotient & Remainder(x=w129, y=w128) -> (x-y*floor(x/y)=w122:i32)  [unwired: 1 out]
                    n49 = control-ref of="Abort AllStage"() -> (w124:refnum<vi>)
                    n50 = call "Defocus and Spherical Comp V2.vi"("Spherical Step"=w120, "Defocus Step"=w121, "Step #"=w122) -> ()  [unwired: 1 in]
                    n51 = call "Piston Comp.vi"("Abort"=w124, "Step Size"=w127, "Step #"=w122, "Original Position"=w126, "Action"=enum16{"MOVE", "BACK TO ORIGINE"}."MOVE") -> ("position"=w123:dbl)  [unwired: 5 in]
                    n52 = property on="Position (µm)" class="DigNum (strict)"("Value"=w123) -> ()  [unwired: 2 in, 2 out]
                  }
                }
              }
            }
            n53 = call "Stage_position_ae.vi"("StageID"="M686", "Enum"=w68) -> ("Position Out"=w78:dbl[])  [unwired: 8 in, 1 out]
            n54 = call "Stage_position_ae.vi"("StageID"="M227", "Enum"=w68) -> ("Position Out"=w85:dbl[])  [unwired: 8 in, 1 out]
            n55 = call "Stage_position_ae.vi"("StageID"="N664", "Enum"=w68) -> ("Position Out"=w71:dbl[])  [unwired: 8 in, 1 out]
            n56 = call "Stage_position_ae.vi"("StageID"="P841", "Enum"=w68) -> ("Position Out"=w92:dbl[])  [unwired: 8 in, 1 out]
            n57 = call "Stage_position_ae.vi"("StageID"="P612", "Enum"=w68) -> ("Position Out"=w69:dbl[])  [unwired: 8 in, 1 out]
            n58 = Index Array(array=w71, index=0) -> (element=w88:dbl)
            n59 = Index Array(array=w92, index=0) -> (element=w65:dbl)
            n60 = Index Array(array=w69, index #1=0 ("index"), index #2=1 ("index"), index #3=2 ("index")) -> (element #1=w98:dbl, element #2=w95:dbl, element #3=w93:dbl)
            n61 = Index Array(array=w78, index #1=0 ("index"), index #2=1 ("index")) -> (element #1=w75:dbl, element #2=w74:dbl)
            n62 = Index Array(array=w85, index #1=0 ("index"), index #2=1 ("index"), index #3=2 ("index")) -> (element #1=w82:dbl, element #2=w81:dbl, element #3=w80:dbl)
            n63 = property on="Position (µm)" class="DigNum (strict)"("Value"=w65) -> ()  [unwired: 2 in, 2 out]
            n64 = property on="Position (mm)" class="DigNum (strict)"("Value"=w88) -> ()  [unwired: 2 in, 2 out]
            n65 = property on="X" class="DigNum (strict)"("Value"=w98) -> ()  [unwired: 2 in, 2 out]
            n66 = property on="Y" class="DigNum (strict)"("Value"=w95) -> ()  [unwired: 2 in, 2 out]
            n67 = property on="X" class="DigNum (strict)"("Value"=w75) -> ()  [unwired: 2 in, 2 out]
            n68 = property on="MM 1" class="DigNum (strict)"("Value"=w82) -> ()  [unwired: 2 in, 2 out]
            n69 = property on="MM 2" class="DigNum (strict)"("Value"=w81) -> ()  [unwired: 2 in, 2 out]
            n70 = property on="Z Position" class="DigNum (strict)"("Value"=w93) -> ()  [unwired: 2 in, 2 out]
            n71 = property on="Y" class="DigNum (strict)"("Value"=w74) -> ()  [unwired: 2 in, 2 out]
            n72 = property on="MM 3" class="DigNum (strict)"("Value"=w80) -> ()  [unwired: 2 in, 2 out]
          }
          frame True {
            w130 = T25."Disabled and Grayed Out" ("Disabled")
            w131 = FALSE ("SLM")
            w134 = enum16{"WRITE", "READ", "HOME", "SAVE HOME"}."SAVE HOME" ("Enum")
            w146 = FALSE ("Upper Shutter")
            n73 = local read "Image Acquisition Parameters"() -> (w153:T19)
            n74 = local read "Laser Controls"() -> (w151:T18)
            n75 = local read "Detectors"() -> (w150:T17)
            n76 = Bundle("Upper Shutter"=w146, "Upper Shutter"=w146) -> (w147:T32)  [unwired: 1 in]
            n77 = property on="Shutters" class="Clust (strict)"("Value"=w147) -> ()  [unwired: 2 in, 2 out]
            n78 = call "Image Aquisition Param Ctrl_AE.vi"("Action"=enum16{"READ", "WRITE"}."WRITE", "Image Acquisition Parameters In"=w153) -> ()  [unwired: 9 in, 1 out]
            n79 = call "Detectors Crl_AE.vi"("Action"=enum16{"READ", "WRITE"}."WRITE", "Detectors Parameters In"=w150) -> ()  [unwired: 9 in, 1 out]
            n80 = call "LASERs_ Crl_AE.vi"("Action"=enum16{"READ", "WRITE"}."WRITE", "Laser Parameters In"=w151) -> ()  [unwired: 9 in, 1 out]
            n81 = property on="Stages" class="Clust (strict)"() -> ("Controls[]"=w148:refnum<vi>[])  [unwired: 2 in, 2 out]
            n82 = for {
              tunnel: w148 -> [w158] mode=indexing
              n83 = property class="Ctl"(reference=w158) -> ("Label.Text"=w156:string, "Value"=w160:variant)  [unwired: 1 in, 2 out]
              n84 = Variant To Data(type=TRUE, Variant=w160) -> (data=w157:bool)  [unwired: 1 in, 1 out]
              n85 = call "All_Stages_Aloha.vi"("Aloha"=w157, "Stage ID"=w156) -> ("Position Out"=w155:dbl[])  [unwired: 9 in]
              n86 = case shown="\"M686\"" w156 {
                tunnel: w155 -> [_ w167 w175 w182 w191 w202 w212]
                frame "0", Default {
                }
                frame "M227" {
                  w171 = FALSE
                  n87 = Index Array(array=w167, index #1=0 ("index"), index #2=1 ("index"), index #3=2 ("index")) -> (element #1=w163:dbl, element #2=w162:dbl, element #3=w161:dbl)
                  n88 = Bundle(w171, w171, 0.0, "Numeric"=w163, "Numeric"=w162, "Numeric"=w161) -> (w169:T33)  [unwired: 1 in]
                  n89 = To Variant(anything=w169) -> (Variant=w168:variant)
                  n90 = property on="Sample Z Coarse - M227" class="Clust"("Value"=w168) -> ()  [unwired: 2 in, 2 out]
                }
                frame "N664" {
                  w172 = FALSE
                  w178 = FALSE ("Down_N664")
                  n91 = Index Array(array=w175, index=0) -> (element=w176:dbl)
                  n92 = Bundle("Down_N664"=w178, "Down_N664"=w178, "Step Size (um)"=1.0, "Numeric"=w176, w172, w172) -> (w174:T34)  [unwired: 1 in]
                  n93 = To Variant(anything=w174) -> (Variant=w173:variant)
                  n94 = property on="Upper Objective Z - N664" class="Clust"("Value"=w173) -> ()  [unwired: 2 in, 2 out]
                }
                frame "P612" {
                  w190 = FALSE
                  n95 = Index Array(array=w182, index #1=0, index #2=1, index #3=2 ("index")) -> (element #1=w187:dbl, element #2=w185:dbl, element #3=w180:dbl)
                  n96 = Bundle(w190, w190, w190, w190, w190, 1.0, "Numeric"=w187, "Numeric"=w185) -> (w186:T35)  [unwired: 1 in]
                  n97 = To Variant(anything=w186) -> (Variant=w181:variant)
                  n98 = property on="Bottom Objective XY - P612" class="Clust"("Value"=w181) -> ()  [unwired: 2 in, 2 out]
                  n99 = property on="Z Position" class="DigNum (strict)"("Value"=w180) -> ()  [unwired: 2 in, 2 out]
                }
                frame "M686" {
                  w200 = FALSE
                  n100 = Index Array(array=w191, index #1=0, index #2=1) -> (element #1=w195:dbl, element #2=w194:dbl)
                  n101 = Bundle(w200, w200, w200, w200, w200, "Numeric"=w195, "Numeric"=w194, 1.0) -> (w198:T36)  [unwired: 1 in]
                  n102 = To Variant(anything=w198) -> (Variant=w196:variant)
                  n103 = property on="Sample Stage XY - M686" class="Clust"("Value"=w196) -> ()  [unwired: 2 in, 2 out]
                  n104 = call "M686_timer.vi"("Reset"=TRUE) -> ()  [unwired: 1 out]
                }
                frame "P841" {
                  n105 = Index Array(array=w202, index=0) -> (element=w201:dbl)
                  n106 = property on="Position (µm)" class="DigNum (strict)"("Value"=w201) -> ()  [unwired: 2 in, 2 out]
                }
                frame "ASI" {
                  w208 = FALSE
                  n107 = Add Array Elements(numeric array=w212) -> (sum=w214:dbl)
                  n108 = Index Array(array=w212, index #1=0 ("index"), index #2=1 ("index")) -> (element #1=w207:dbl, element #2=w206:dbl)
                  n109 = Divide(x=w214, y=2000.0) -> ()  [unwired: 1 out]
                  n110 = Bundle By Name(cluster=T7 {"Up ASI"=FALSE, "Down ASI"=FALSE, "Step Size (um)"=0.001, "Z (um)"=0.001, "F (um)"=0.001, "Velocity"=0.001} ("Cavity Translation Z - ASI"), "Up ASI"=w208, "Down ASI"=w208, "Step Size (um)"=1.0, "Z (um)"=w207, "F (um)"=w206, "Velocity"=0.1) -> (w204:T7)
                  n111 = To Variant(anything=w204) -> (Variant=w205:variant)
                  n112 = property on="Cavity Translation Z - ASI" class="Clust"("Value"=w205) -> ()  [unwired: 2 in, 2 out]
                }
              }
            }
            n113 = call-poly <vilib>:"Read From Spreadsheet File.vi"("format (%.3f)"="%.4f", "number of rows (all:-1)"=1, "file path (dialog if empty)"=path "C:/Users/ED STED/Documents/Test Control Software/Host VIs/Stages/Stage Positions/home position.csv") -> ("first row"=w143:dbl[])  [unwired: 4 in, 4 out]
            n114 = Index Array(array=w143, index #1=0 ("index"), index #2=1 ("index")) -> (element #1=w139:dbl, element #2=w140:dbl)
            n115 = Build Array(w139) -> (w138:dbl[])
            n116 = Build Array(w140) -> (w136:dbl[])
            n117 = call "Stage_position_ae.vi"("Position In"=w138, "StageID"="P541", "Enum"=w134) -> ()  [unwired: 7 in, 2 out]
            n118 = call "Stage_position_ae.vi"("Position In"=w136, "StageID"="N664", "Enum"=w134) -> ()  [unwired: 7 in, 2 out]
            n119 = local write "Sequence"(w131) -> ()
            n120 = local write "Focus Lock"(w131) -> ()
            n121 = local write "SLM"(w131) -> ()
            n122 = local write "Timing"(w131) -> ()
            n123 = local write "DM"(w131) -> ()
            n124 = local write "Camera"(w131) -> ()
            n125 = property on="Sequence Cluster" class="Clust"("DisabledEnum"=w130) -> ()  [unwired: 2 in, 2 out]
            n126 = property on="Sequence List" class="RadioBtnsControl (strict)"("DisabledEnum"=w130) -> ()  [unwired: 2 in, 2 out]
            n127 = property on="Seq 3" class="Bool (strict)"("DisabledEnum"=w130) -> ()  [unwired: 2 in, 2 out]
            n128 = property on="Seq 1" class="Bool (strict)"("DisabledEnum"=w130) -> ()  [unwired: 2 in, 2 out]
            n129 = property on="Seq 2" class="Bool (strict)"("DisabledEnum"=w130) -> ()  [unwired: 2 in, 2 out]
            n130 = property on="Seq 4" class="Bool (strict)"("DisabledEnum"=w130) -> ()  [unwired: 2 in, 2 out]
            n131 = call "Frame Counter.vi"("Action"=Counter_Action."Zero") -> ()  [unwired: 1 out]
          }
        }
        n132 = local read "Capture"() -> (w56:bool)
        n133 = And(x=w57, y=w56) -> (x .and. y?=w54:bool)
        n134 = case shown="True" w54 {
          tunnel: w55 -> [_ w220]
          frame False {
          }
          frame True {
            w218 = T25."Enabled" ("Disabled")
            n135 = local write "Capture"(FALSE ("Capture")) -> ()
            n136 = call "Frame Counter.vi"("Action"=Counter_Action."Zero") -> ()  [unwired: 1 out]
            n137 = Enqueue Element(queue=w220, element="Stop Acquisition" ("f")) -> ()  [unwired: 2 in, 3 out]
            n138 = property on="Live" class="Bool (strict)"("DisabledEnum"=w218) -> ()  [unwired: 2 in, 2 out]
            n139 = property on="Exit" class="Bool"("DisabledEnum"=w218) -> ()  [unwired: 2 in, 2 out]
          }
        }
      }
      event Value Change {
        w229 = Standard_Action."Read" ("Action")
        n140 = event-data() -> ("NewVal"=w230:T1, "OldVal"=w235:T1)  [unwired: 1 in]
        n141 = Not Equal?(x=w230, y=w235) -> (x != y?=w234:T37)
        n142 = Unbundle By Name(w230) -> ("Enable"=w233:bool)
        n143 = Unbundle By Name(w234) -> ("Enable"=w232:bool)
        n144 = call "Pixel Value (-1 to 1) DUAL AE.vi"("Action"=w229) -> ("Pixel Value (-1 to 1) Out"=w222:dbl[][])  [unwired: 14 in]
        n145 = call "Mirror_Mode_DUAL_AE.vi"("Action"=w229) -> ("Mirror Modes Out"=w228:T38)  [unwired: 14 in]
        n146 = And(x=w233, y=w232) -> (x .and. y?=w231:bool)
        n147 = case shown="False" w231 {
          tunnel: w230 -> [w239 w248]
          tunnel: w222 -> [w236 w241]
          tunnel: w228 -> [w240 w242]
          tunnel: [w237 w243] -> w227
          tunnel: [w239 w243] -> w225
          tunnel: [w236 w241] -> w224
          tunnel: [w240 w242] -> w223
          frame False {
            n148 = Bundle By Name(cluster=w239, "Origin (um)"=0.0) -> (w237:T1)
          }
          frame True {
            n149 = call "AE_AllStages_Action V2.vi"("Stage ID"="P841" ("StageID"), "Action"=StageStates."MVR") -> ("Position Out"=w244:dbl[])  [unwired: 7 in, 2 out]
            n150 = Index Array(array=w244, index=0) -> (element=w247:dbl)
            n151 = Bundle By Name(cluster=w248, "Origin (um)"=w247) -> (w243:T1)
          }
        }
        n152 = local write "z Comp."(w227) -> ()
        n153 = call "AO AE.vi"("Mirror Modes In"=w223, "DM Value Input"=w224, "Z Comp. Input"=w225, "Action"=enum16{"READ", "WRITE"}."WRITE") -> ()  [unwired: 5 in, 3 out]
      }
      event "Capture": Value Change {
        w255 = FALSE ("element")
        n154 = event-data() -> ("CtlRef"=w263:refnum<vi>, "NewVal"=w252:variant)  [unwired: 1 in]
        n155 = call "Detectors Crl_AE.vi"() -> ("Detectors Parameters Out"=w261:T17)  [unwired: 11 in]
        n156 = Unbundle By Name(w261) -> ("PMT"=w260:bool, "Far Red (685/40 nm)"=w259:bool, "Orange (624/40 nm)"=w258:bool, "Green (525/50 nm)"=w257:bool, "Sum All"=w256:bool)
        n157 = Variant To Data(type=TRUE, Variant=w252) -> (data=w250:bool)  [unwired: 1 in, 1 out]
        n158 = Build Array(w260, w259, w258, w257, w256, w255, w255, w255) -> (w254:bool[])
        n159 = Boolean Array To Number(Boolean array=w254) -> (number=w253:u32)
        n160 = case shown="1, Default" w253 {
          tunnel: w264 -> [_ w275]
          tunnel: w263 -> [_ w274]
          tunnel: w262 -> [_ w270]
          tunnel: w250 -> [_ w269]
          frame 0 {
            w266 = FALSE ("Live")
            n161 = call "Display Message to User"() -> ()  [unwired: 10 in, 2 out]
            n162 = local write "Capture"(w266) -> ()
            n163 = local write "Live"(w266) -> ()
          }
          frame 1, Default {
            n164 = Not(x=w269) -> (.not. x?=w272:bool)
            n165 = property class="Bool (strict)"(reference=w274) -> ("Label.Text"=w271:string)  [unwired: 1 in, 2 out]
            n166 = Send Notification(notification=w272, notifier=w270) -> ()  [unwired: 1 in, 2 out]
            n167 = Select(t=w271, s=w269, f="Stop Acquisition") -> (s? t:f=w268:string)
            n168 = case shown="\"Capture\"" w271 {
              tunnel: w269 -> [_ w279 w295]
              tunnel: w268 -> [w276 w277 w294]
              tunnel: [w276 w277 w293] -> w267
              frame "False", Default {
              }
              frame "Live" {
                n169 = case shown="True" w279 {
                  tunnel: [T25."Enabled" ("Disabled") T25."Disabled and Grayed Out" ("Disabled")] -> w278
                  frame False {
                    n170 = call "Frame Counter.vi"("Action"=Counter_Action."Zero") -> ()  [unwired: 1 out]
                  }
                  frame True {
                    n171 = call "AO AE.vi"("Action"=enum16{"READ", "WRITE"}."READ") -> ("DM Value Output"=w284:dbl[][], "Z Comp. Output"=w283:T1)  [unwired: 8 in, 1 out]
                    n172 = Unbundle By Name(w283) -> ("Enable"=w282:bool)
                    n173 = call "Frame Counter.vi"("Action"=Counter_Action."Zero") -> ()  [unwired: 1 out]
                    n174 = case shown="True" w282 {
                      tunnel: w284 -> [_ w289]
                      tunnel: w283 -> [_ w288]
                      frame False {
                      }
                      frame True {
                        n175 = call "Mirror_Mode_DUAL_AE.vi"("Action"=Standard_Action."Read") -> ("Mirror Modes Out"=w291:T38)  [unwired: 14 in]
                        n176 = call "AO AE.vi"("Mirror Modes In"=w291, "DM Value Input"=w289, "Z Comp. Input"=w288, "Action"=enum16{"READ", "WRITE"}."WRITE") -> ()  [unwired: 5 in, 3 out]
                      }
                    }
                  }
                }
                n177 = property on="Capture" class="Bool (strict)"("DisabledEnum"=w278) -> ()  [unwired: 2 in, 2 out]
                n178 = property on="Exit" class="Bool"("DisabledEnum"=w278) -> ()  [unwired: 2 in, 2 out]
              }
              frame "Capture" {
                n179 = case shown="True" w295 {
                  tunnel: [T25."Enabled" ("Disabled") T25."Disabled and Grayed Out" ("Disabled")] -> w296
                  tunnel: w294 -> [w297 w310]
                  tunnel: [w297 w309] -> w293
                  frame False {
                    n180 = call "AO AE.vi"("Action"=enum16{"READ", "WRITE"}."READ") -> ("DM Value Output"=w300:dbl[][], "Z Comp. Output"=w299:T1)  [unwired: 8 in, 1 out]
                    n181 = call "Frame Counter.vi"("Action"=Counter_Action."Zero") -> ()  [unwired: 1 out]
                    n182 = Unbundle By Name(w299) -> ("Enable"=w298:bool)
                    n183 = case shown="True" w298 {
                      tunnel: w300 -> [_ w305]
                      tunnel: w299 -> [_ w304]
                      frame False {
                      }
                      frame True {
                        n184 = call "Mirror_Mode_DUAL_AE.vi"("Action"=Standard_Action."Read") -> ("Mirror Modes Out"=w307:T38)  [unwired: 14 in]
                        n185 = call "AO AE.vi"("Mirror Modes In"=w307, "DM Value Input"=w305, "Z Comp. Input"=w304, "Action"=enum16{"READ", "WRITE"}."WRITE") -> ()  [unwired: 5 in, 3 out]
                      }
                    }
                  }
                  frame True {
                    n186 = local read "Sequence"() -> (w311:T14)
                    n187 = case shown="True" w311 {
                      tunnel: w310 -> [w314 w317]
                      tunnel: [w314 w316] -> w309
                      frame False {
                      }
                      frame True {
                        n188 = call "Seq AE.vi"("Action"=enum16{"READ", "BUILD", "WRITE", "DELETE"}."READ") -> ("Array"=w315:T39)  [unwired: 8 in]
                        n189 = Array Size(array=w315) -> (size(s)=w320:i32)
                        n190 = Equal?(x=w320, y=0) -> (x = y?=w318:bool)
                        n191 = case shown="False" w318 {
                          tunnel: ["Sequence" ("f") w330] -> w316
                          tunnel: w317 -> [_ w330]
                          tunnel: w315 -> [w329 _]
                          frame False {
                            w323 = enum16{"READ", "WRITE"}."WRITE" ("Action")
                            n192 = Index Array(array=w329, index=0) -> (element=w327:T40)
                            n193 = Unbundle By Name(w327) -> ("Detectors Parameters Out"=w326:T17, "Laser Parameters Out"=w325:T18, "Image Acquisition Parameters Out"=w324:T19)
                            n194 = call "Detectors Crl_AE.vi"("Action"=w323, "Detectors Parameters In"=w326) -> ()  [unwired: 9 in, 1 out]
                            n195 = call "LASERs_ Crl_AE.vi"("Action"=w323, "Laser Parameters In"=w325) -> ()  [unwired: 9 in, 1 out]
                            n196 = call "Image Aquisition Param Ctrl_AE.vi"("Action"=w323, "Image Acquisition Parameters In"=w324) -> ()  [unwired: 9 in, 1 out]
                          }
                          frame True {
                          }
                        }
                      }
                    }
                    n197 = call "Frame Counter.vi"("Action"=Counter_Action."Zero") -> ()  [unwired: 1 out]
                  }
                }
                n198 = property on="Live" class="Bool (strict)"("DisabledEnum"=w296) -> ()  [unwired: 2 in, 2 out]
                n199 = property on="Exit" class="Bool"("DisabledEnum"=w296) -> ()  [unwired: 2 in, 2 out]
              }
            }
            n200 = Enqueue Element(queue=w275, element=w267) -> ()  [unwired: 2 in, 3 out]
          }
        }
      }
      event "Shutters": Value Change {
        n201 = event-data() -> ("CtlRef"=w334:refnum<vi>, "NewVal"=w333:variant, "OldVal"=w332:variant)  [unwired: 1 in]
        n202 = property class="Clust"(reference=w334) -> ("Label.Text"=w331:string)  [unwired: 1 in, 2 out]
        n203 = case shown="\"Shutters\"" w331 {
          tunnel: w333 -> [_ w350 _ _ _]
          tunnel: w332 -> [_ w348 _ _ _]
          frame Default {
          }
          frame "Image Acquisition Parameters" {
            n204 = Variant To Data(type="Image Acquisition Parameters", Variant=w350) -> (data=w347:T19)  [unwired: 1 in, 1 out]
            n205 = Variant To Data(type=w347, Variant=w348) -> (data=w346:T19)  [unwired: 1 in, 1 out]
            n206 = Not Equal?(x=w347, y=w346) -> (x != y?=w371:T41)
            n207 = Unbundle By Name(w371) -> ("Image Dimension (um)"=w356:bool[], "Image Format"=w354:bool, "Pixel Size (nm)"=w355:bool[], "Scan Mode"=w337:bool)
            n208 = Or Array Elements(Boolean array=w356) -> (logical OR=w360:bool)
            n209 = Or Array Elements(Boolean array=w355) -> (logical OR=w359:bool)
            n210 = Build Array(w360, w354, w359) -> (w358:bool[])
            n211 = Boolean Array To Number(Boolean array=w358) -> (number=w357:u32)
            n212 = case shown="1, 2" w357 {
              tunnel: w356 -> [_ w421 _]
              tunnel: w347 -> [w409 w414 w429]
              tunnel: [w409 w412 w427] -> w353
              tunnel: w355 -> [_ _ w426]
              tunnel: [w408 w411 w425] -> w352
              tunnel: [w407 w410 w424] -> w339
              frame 0, Default {
                n213 = Unbundle By Name(w409) -> ("Image Dimension (um)"=w408:dbl[], "Scan Mode"=w407:enum16{"XY", "XZ", "YZ", "XYZ"})
              }
              frame 1, 2 {
                # "Image Dimension or Format Change"
                n214 = Unbundle By Name(w414) -> ("Image Dimension (um)"=w420:dbl[], "Image Format"=w418:u16, "Scan Mode"=w410:enum16{"XY", "XZ", "YZ", "XYZ"})
                n215 = for {
                  tunnel: w421 -> [w423] mode=indexing
                  tunnel: w420 -> [w422] mode=indexing
                  tunnel: [w422] -> w419
                  stop <- w423 stop-if-true
                }
                n216 = To Double Precision Float(number=w418) -> (double precision float=w417:dbl)
                n217 = Build Array(w419, w419) -> (w411:dbl[])
                n218 = Divide(x=w411, y=w417) -> (x/y=w416:dbl[])
                n219 = Multiply(x=w416, y=1000.0) -> (x*y=w413:dbl[])
                n220 = Bundle By Name(cluster=w414, "Image Dimension (um)"=w411, "Pixel Size (nm)"=w413) -> (w412:T19)
              }
              frame 4 {
                # "Pixel Size Change"
                n221 = Unbundle By Name(w429) -> ("Pixel Size (nm)"=w435:dbl[], "Image Format"=w433:u16, "Scan Mode"=w424:enum16{"XY", "XZ", "YZ", "XYZ"})
                n222 = for {
                  tunnel: w426 -> [w437] mode=indexing
                  tunnel: w435 -> [w436] mode=indexing
                  tunnel: [w436] -> w434
                  stop <- w437 stop-if-true
                }
                n223 = Build Array(w434, w434) -> (w428:dbl[])
                n224 = To Double Precision Float(number=w433) -> (double precision float=w432:dbl)
                n225 = Multiply(x=w428, y=w432) -> (x*y=w431:dbl[])
                n226 = Multiply(x=w431, y=0.001) -> (x*y=w425:dbl[])
                n227 = Bundle By Name(cluster=w429, "Pixel Size (nm)"=w428, "Image Dimension (um)"=w425) -> (w427:T19)
              }
            }
            n228 = And(x=w337, y="Follow Cursor") -> (x .and. y?=w336:bool)
            n229 = case shown="True" w336 {
              tunnel: w339 -> [_ w381]
              frame False {
              }
              frame True {
                n230 = Not Equal?(x=w381, y=enum16{"XY", "XZ", "YZ", "XYZ"}."XZ") -> (x != y?=w379:bool)
                n231 = case shown="True" w379 {
                  frame False {
                    n232 = call "Y Slice.vi"() -> ("Y position"=w389:dbl)  [unwired: 1 in]
                    n233 = Build Array(0.0 ("element"), w389) -> (w387:dbl[])
                    n234 = call "AllStage_Limits_Array.vi"("Step(um)/Position(units)"=w387, "Axis"=bool[] [TRUE, TRUE, TRUE], "Stage ID"="M686", "MOVE/MVR"=enum16{"MOVE", "MVR"}."MVR") -> ("Positions"=w383:dbl[], "Boolean Array"=w384:bool[], "Stage ID"=w385:string)  [unwired: 4 in, 1 out]
                    n235 = call "AE_AllStages_Action V2.vi"("Velocity"=0.0, "Positions"=w383, "Axis"=w384, "Stage ID"=w385, "Action"=StageStates."MVR") -> ()  [unwired: 4 in, 3 out]
                  }
                  frame True {
                    n236 = call "Z Slice.vi"() -> ("Z position"=w403:dbl)  [unwired: 1 in]
                    n237 = call "Manual Controls Action Engine.vi"("Action"=enum16{"Read", "Write"}."Read") -> ("Manual Controls Out"=w398:T21)  [unwired: 14 in]
                    n238 = Multiply(x=w403, y=327.68) -> (x*y=w405:dbl)
                    n239 = Round To Nearest(number=w405) -> (nearest integer value=w404:dbl)
                    n240 = Unbundle By Name(w398) -> ("Z Axis Voltage (I16)"=w401:i16)
                    n241 = To Word Integer(number=w404) -> (16bit integer=w400:i16)
                    n242 = Add(x=w401, y=w400) -> (x+y=w399:i16)
                    n243 = Bundle By Name(cluster=w398, "Z Axis Voltage (I16)"=w399) -> (w397:T21)
                    n244 = call "Manual Controls Action Engine.vi"("Action"=enum16{"Read", "Write"}."Write", "Manual Controls In"=w397) -> ("Manual Controls Out"=w395:T21)  [unwired: 13 in]
                    n245 = call "FPGA-7842R-Control V2.vi"("Action"=FPGA-7842R-Reference."Stage Control", "Manual Controls"=w395, "Initialize"=TRUE) -> ()  [unwired: 11 in, 2 out]
                  }
                }
              }
            }
            n246 = Index Array(array=w352, index=0) -> (element=w376:dbl)
            n247 = Not Equal?(x=enum16{"XY", "XZ", "YZ", "XYZ"}."YZ" ("y"), y=w339) -> (x != y?=w361:bool)
            n248 = call "Res Mirror um to Volts.vi"("Image Size (um)"=w376) -> ("Voltage (V)"=w340:dbl)
            n249 = Select(t=15780.0, s=w361, f=200.0) -> (s? t:f=w364:dbl)
            n250 = In Range and Coerce(upper limit=5.0, x=w340, lower limit=0.0) -> (coerced(x)=w342:dbl)  [unwired: 1 out]
            n251 = call "Scan Parameters Action Engine.vi"("Action"=enum16{"Read", "Write"}."Read") -> ("Scan Parameters OUT"=w343:T20)  [unwired: 14 in]
            n252 = Bundle By Name(cluster=w343, "Fast_Ax_Amp_V"=w342) -> (w341:T20)
            n253 = Bundle By Name(cluster=w353, "Fast Axis Frequency (Hz)"=w364) -> (w363:T19)
            n254 = call "Volts to I16.vi"("Voltage (V)"=w342) -> ("I16"=w375:i16)  [unwired: 13 in, 1 out]
            n255 = call "Scan Parameters Action Engine.vi"("Action"=enum16{"Read", "Write"}."Write", "Scan Parameters IN"=w341) -> ()  [unwired: 13 in, 1 out]
            n256 = call "Manual Controls Action Engine.vi"("Action"=enum16{"Read", "Write"}."Read") -> ("Manual Controls Out"=w369:T21)  [unwired: 14 in]
            n257 = Bundle By Name(cluster=w369, "Res Mirror Amp (I16)"=w375, "Res Mirror Mute"=w361) -> (w367:T21)
            n258 = call "Image Aquisition Param Ctrl_AE.vi"("Action"=enum16{"READ", "WRITE"}."WRITE", "Image Acquisition Parameters In"=w363) -> ()  [unwired: 9 in, 1 out]
            n259 = call "FPGA-7842R-Control V2.vi"("Action"=FPGA-7842R-Reference."Set Res Mirror", "Manual Controls"=w367, "Initialize"=TRUE) -> ()  [unwired: 11 in, 2 out]
            n260 = call "Manual Controls Action Engine.vi"("Action"=enum16{"Read", "Write"}."Write", "Manual Controls In"=w367) -> ()  [unwired: 13 in, 1 out]
          }
          frame "Detectors" {
            n261 = call "Detectors Crl_AE.vi"("Action"=enum16{"READ", "WRITE"}."WRITE", "Detectors Parameters In"="Detectors") -> ()  [unwired: 9 in, 1 out]
          }
          frame "Laser Controls" {
            w452 = FALSE ("element")
            n262 = Unbundle By Name("Laser Controls") -> ("STED"=w458:bool, "650 nm"=w455:bool, "590 nm"=w456:bool, "485 nm"=w457:bool, "STED Power (V)"=w449:dbl, "Manual Control"=w441:bool)
            n263 = local read "Live"() -> (w444:T14)
            n264 = call "LASERs_ Crl_AE.vi"("Action"=enum16{"READ", "WRITE"}."WRITE", "Laser Parameters In"="Laser Controls") -> ()  [unwired: 9 in, 1 out]
            n265 = Or(x=w444, y=w441) -> (x .or. y?=w443:T14)
            n266 = In Range and Coerce(upper limit=10.0, x=w449, lower limit=0.0) -> (coerced(x)=w446:dbl)  [unwired: 1 out]
            n267 = Build Array(w458, w455, w456, w457, w452, w452, w452, w452) -> (w454:bool[])
            n268 = case shown="True" w443 {
              tunnel: "Laser Controls" -> [_ w472]
              frame False {
              }
              frame True {
                n269 = call "FPGA-7842R-Control V2.vi"("Action"=FPGA-7842R-Reference."Laser Control", "Laser Controls"=w472, "Initialize"=TRUE) -> ()  [unwired: 11 in, 2 out]
              }
            }
            n270 = Boolean Array To Number(Boolean array=w454) -> (number=w453:u32)
            n271 = To Unsigned Byte Integer(number=w453) -> (unsigned 8bit integer=w451:u8)
            n272 = call "U8_To_U32.vi"("U8 IN"=w451) -> ("U32 OUT"=w450:u32)  [unwired: 13 in, 1 out]
            n273 = call "Volts to I16.vi"("Voltage (V)"=w446) -> ("I16"=w445:i16)  [unwired: 13 in, 1 out]
            n274 = case shown="False" w441 {
              tunnel: "Laser Controls" -> [w470 _]
              frame False {
                n275 = Unbundle By Name(w470) -> ("650 nm"=w467:bool, "590 nm"=w466:bool, "485 nm"=w465:bool)
                n276 = call "Detectors Crl_AE.vi"("Action"=enum16{"READ", "WRITE"}."READ") -> ("Detectors Parameters Out"=w468:T17)  [unwired: 10 in]
                n277 = Bundle By Name(cluster=w468, "Far Red (685/40 nm)"=w467, "Orange (624/40 nm)"=w466, "Green (525/50 nm)"=w465) -> (w464:T17)
                n278 = call "Detectors Crl_AE.vi"("Action"=enum16{"READ", "WRITE"}."WRITE", "Detectors Parameters In"=w464) -> ()  [unwired: 9 in, 1 out]
              }
              frame True {
              }
            }
            n279 = call "Scan Parameters Action Engine.vi"("Action"=enum16{"Read", "Write"}."Read") -> ("Scan Parameters OUT"=w461:T20)  [unwired: 14 in]
            n280 = Bundle By Name(cluster=w461, "Laser_States _U32"=w450, "775_AOM_Volt_I16"=w445) -> (w459:T20)
            n281 = call "Scan Parameters Action Engine.vi"("Action"=enum16{"Read", "Write"}."Write", "Scan Parameters IN"=w459) -> ()  [unwired: 13 in, 1 out]
          }
          frame "Shutters" {
            n282 = Unbundle By Name("Shutters") -> ("Upper Shutter"=w484:bool, "Lower Shutter"=w483:bool)
            n283 = Not(x=w484) -> (.not. x?=w475:bool)
            n284 = Not(x=w483) -> (.not. x?=w474:bool)
            n285 = call "Manual Controls Action Engine.vi"("Action"=enum16{"Read", "Write"}."Read") -> ("Manual Controls Out"=w479:T21)  [unwired: 14 in]
            n286 = Bundle By Name(cluster=w479, "Upper Shutter"=w475, "Lower Shutter"=w474) -> (w476:T21)
            n287 = call "Manual Controls Action Engine.vi"("Action"=enum16{"Read", "Write"}."Write", "Manual Controls In"=w476) -> ()  [unwired: 13 in, 1 out]
            n288 = call "FPGA-7842R-Control V2.vi"("Action"=FPGA-7842R-Reference."Shutter Control", "Manual Controls"=w476, "Initialize"=TRUE) -> ()  [unwired: 11 in, 2 out]
          }
        }
      }
      event Value Change {
        # "For P541 - Sample Z - Converting from Step in µm to I16 is as follows. We have (Step µw)*(10 V / 100 µm)*(32768 I16 / 10 V) = (Step µm)*(32768 I16 / 100 µm) = (Step µm)*(327.68 I16/µm)"
        n289 = event-data() -> ("CtlRef"=w498:refnum<vi>, "OldVal"=w496:variant, "NewVal"=w497:variant)  [unwired: 1 in]
        n290 = local write "Abort AllStage"(FALSE ("Abort AllStage")) -> ()
        n291 = property class="Clust"(reference=w498) -> ("Label.Text"=w495:string)  [unwired: 1 in, 2 out]
        n292 = case shown="\"Sample Z - P541\"" w495 {
          tunnel: w497 -> [_ w521 w562 w589 w652 w693 w722 w762]
          tunnel: w496 -> [_ w520 w561 w588 w653 w694 w723 w763]
          tunnel: ["" "N664" "ASI" "P612" "P612" "P841" "M227" "M686"] -> w494
          tunnel: [dbl[] [0.0] w512 w554 w577 dbl[] [0.0] w682 w715 w752] -> w493
          tunnel: [bool[] [FALSE] w510 w548 w578 bool[] [FALSE] bool[] [TRUE] w716 w751] -> w492
          tunnel: [enum16{"MOVE", "MVR"}."MVR" ("MOVE/MVR") w509 w551 w580 enum16{"MOVE", "MVR"}."MVR" ("MOVE/MVR") w685 w708 w754] -> w491
          tunnel: [0.0 ("Step Size (um)") 0.5 ("Step Size (um)") w553 0.0 ("Velocity") 0.0 ("Velocity") 10000.0 ("Velocity") 0.0 ("Velocity") 0.0 ("Velocity")] -> w487
          tunnel: [StageStates."MVR" ("Action") w507 w552 w581 StageStates."POSITION" ("Action") w686 w712 w755] -> w485
          frame Default {
          }
          frame "Upper Objective Z - N664" {
            n293 = call "N664_Ctrl_Index.vi"("OldVal"=w520, "NewVal"=w521) -> ("Control Ref OUT"=w519:refnum<vi>, "N664 Out"=w517:T6)  [unwired: 12 in]
            n294 = property class="Ctl"(reference=w519) -> ("Label.Text"=w518:string)  [unwired: 1 in, 2 out]
            n295 = Unbundle By Name(w517) -> ("Step Size (um)"=w516:dbl, "Position (mm)"=w515:dbl)
            n296 = case shown="\"Home\"" w518 {
              tunnel: w516 -> [_ w526 w529 _ _ _]
              tunnel: [0.0 ("Step Size (um)") w525 w529 w534 w536 w541] -> w513
              tunnel: w515 -> [_ _ _ w534 w536 _]
              tunnel: [enum16{"MOVE", "MVR"}."MVR" ("MOVE/MVR") enum16{"MOVE", "MVR"}."MVR" ("MOVE/MVR") enum16{"MOVE", "MVR"}."MVR" ("MOVE/MVR") enum16{"MOVE", "MVR"}."MOVE" ("MOVE/MVR") enum16{"MOVE", "MVR"}."MOVE" ("MOVE/MVR") enum16{"MOVE", "MVR"}."MOVE" ("MOVE/MVR")] -> w509
              tunnel: [StageStates."MVR" ("Action") StageStates."MVR" ("Action") StageStates."MVR" ("Action") StageStates."MOVE" ("Action") StageStates."MOVE" ("Action") StageStates."MOVE" ("Action")] -> w507
              frame Default {
              }
              frame "Up N664" {
                n297 = Negate(x=w526) -> (-x=w525:dbl)
              }
              frame "Down N664" {
              }
              frame "Position (mm)" {
              }
              frame "Save" {
                n298 = Build Array(w536) -> (w535:dbl[])
                n299 = call "Stage_position_ae.vi"("Position In"=w535, "StageID"="N664", "Enum"=enum16{"WRITE", "READ", "HOME", "SAVE HOME"}."SAVE HOME") -> ()  [unwired: 7 in, 2 out]
              }
              frame "Home" {
                n300 = call "Stage_position_ae.vi"("StageID"="N664", "Enum"=enum16{"WRITE", "READ", "HOME", "SAVE HOME"}."HOME") -> ("Position Out"=w543:dbl[])  [unwired: 8 in, 1 out]
                n301 = Index Array(array=w543, index=0) -> (element=w541:dbl)
              }
            }
            n302 = Build Array(w513) -> (w512:dbl[])
            n303 = Build Array(TRUE) -> (w510:bool[])
          }
          frame "Cavity Translation Z - ASI" {
            n304 = call "ASI_Ctrl_Index.vi"("NewVal"=w562, "OldVal"=w561) -> ("ASI out"=w558:T7, "Control Ref OUT"=w560:refnum<vi>)  [unwired: 8 in]
            n305 = property class="Ctl"(reference=w560) -> ("Label.Text"=w559:string)  [unwired: 1 in, 2 out]
            n306 = Unbundle By Name(w558) -> ("Step Size (um)"=w557:dbl, "Z (um)"=w556:dbl, "Velocity"=w553:dbl)
            n307 = case shown="\"Z (um)\"" w559 {
              tunnel: w557 -> [_ w568 w571 _]
              tunnel: w556 -> [_ _ _ w575]
              tunnel: [0.0 ("Z (um)") w568 w572 w575] -> w555
              tunnel: [StageStates."MVR" ("Action") StageStates."MVR" ("Action") StageStates."MVR" ("Action") StageStates."MOVE" ("Action")] -> w552
              tunnel: [enum16{"MOVE", "MVR"}."MVR" ("MOVE/MVR") enum16{"MOVE", "MVR"}."MVR" ("MOVE/MVR") enum16{"MOVE", "MVR"}."MVR" ("MOVE/MVR") enum16{"MOVE", "MVR"}."MOVE" ("MOVE/MVR")] -> w551
              frame Default {
              }
              frame "Up ASI" {
              }
              frame "Down ASI" {
                n308 = Negate(x=w571) -> (-x=w572:dbl)
              }
              frame "Z (um)" {
              }
            }
            n309 = Build Array(w555) -> (w554:dbl[])
            n310 = Build Array(TRUE) -> (w548:bool[])
          }
          frame "Bottom Objective XY - P612" {
            n311 = call "P612_Ctrl_Index.vi"("OldVal"=w588, "NewVal"=w589) -> ("Control out"=w587:refnum<vi>, "P612 out"=w585:T10)  [unwired: 12 in]
            n312 = property class="Ctl"(reference=w587) -> ("Label.Text"=w586:string)  [unwired: 1 in, 2 out]
            n313 = Unbundle By Name(w585) -> ("Step Size (um)"=w584:dbl, "X"=w583:dbl, "Y"=w582:dbl)
            n314 = case shown="\"Up Button\"" w586 {
              tunnel: w584 -> [_ _ w600 w607 w611 w618 _]
              tunnel: w583 -> [_ _ _ _ _ _ w625]
              tunnel: w582 -> [_ _ _ _ _ _ w624]
              tunnel: [StageStates."MVR" ("Action") StageStates."HOME" ("Action") StageStates."MVR" ("Action") StageStates."MVR" ("Action") StageStates."MVR" ("Action") StageStates."MVR" ("Action") StageStates."MOVE" ("Action")] -> w581
              tunnel: [enum16{"MOVE", "MVR"}."MVR" ("MOVE/MVR") enum16{"MOVE", "MVR"}."MVR" ("MOVE/MVR") enum16{"MOVE", "MVR"}."MVR" ("MOVE/MVR") enum16{"MOVE", "MVR"}."MVR" ("MOVE/MVR") enum16{"MOVE", "MVR"}."MVR" ("MOVE/MVR") enum16{"MOVE", "MVR"}."MVR" ("MOVE/MVR") enum16{"MOVE", "MVR"}."MOVE" ("MOVE/MVR")] -> w580
              tunnel: [bool[] [FALSE] bool[] [TRUE, TRUE] bool[] [TRUE, FALSE] bool[] [TRUE, FALSE] bool[] [FALSE, TRUE] bool[] [FALSE, TRUE] bool[] [TRUE, TRUE]] -> w578
              tunnel: [dbl[] [0.0] dbl[] [0.0, 0.0] w599 w606 w613 w620 w626] -> w577
              frame Default {
              }
              frame "Home Button" {
              }
              frame "Up Button" {
                n315 = Build Array(w600, 0.0 ("element")) -> (w599:dbl[])
              }
              frame "Down Button" {
                n316 = Negate(x=w607) -> (-x=w604:dbl)
                n317 = Build Array(w604, 0.0 ("element")) -> (w606:dbl[])
              }
              frame "Left Button" {
                n318 = Build Array(0.0 ("element"), w611) -> (w613:dbl[])
              }
              frame "Right Button" {
                n319 = Negate(x=w618) -> (-x=w617:dbl)
                n320 = Build Array(0.0 ("element"), w617) -> (w620:dbl[])
              }
              frame "X", "Y" {
                n321 = Build Array(w625, w624) -> (w626:dbl[])
              }
            }
          }
          frame "Sample Z - P541" {
            w631 = 327.68 ("y")
            n322 = call "P541_Ctrl_Index.vi"("OldVal"=w653, "NewVal"=w652) -> ("Control out"=w651:refnum<vi>, "P541 Out"=w650:T16)  [unwired: 12 in]
            n323 = Unbundle By Name(w650) -> ("Z Position"=w630:dbl, "Step Size (um)"=w649:dbl)
            n324 = property class="Ctl"(reference=w651) -> ("Label.Text"=w648:string)  [unwired: 1 in, 2 out]
            n325 = call "Manual Controls Action Engine.vi"("Action"=enum16{"Read", "Write"}."Read") -> ("Manual Controls Out"=w639:T21)  [unwired: 14 in]
            n326 = Unbundle By Name(w639) -> ("Z Axis Voltage (I16)"=w642:i16)
            n327 = Multiply(x=w630, y=w631) -> (x*y=w645:dbl)
            n328 = Multiply(x=w649, y=w631) -> (x*y=w647:dbl)
            n329 = Round To Nearest(number=w645) -> (nearest integer value=w634:dbl)
            n330 = Round To Nearest(number=w647) -> (nearest integer value=w633:dbl)
            n331 = To Word Integer(number=w634) -> (16bit integer=w644:i16)
            n332 = To Word Integer(number=w633) -> (16bit integer=w646:i16)
            n333 = case shown="\"Home\"" w648 {
              tunnel: w646 -> [_ w660 w664 _ _ _]
              tunnel: w644 -> [_ _ _ w666 _ _]
              tunnel: w642 -> [w659 w662 w665 _ w671 _]
              tunnel: [w659 w661 w663 w666 w671 w677] -> w638
              tunnel: w631 -> [_ _ _ _ _ w676]
              tunnel: w630 -> [_ _ _ _ w670 _]
              frame Default {
              }
              frame "Step Down" {
                n334 = Subtract(x=w662, y=w660) -> (x-y=w661:i16)
              }
              frame "Step Up" {
                n335 = Add(x=w665, y=w664) -> (x+y=w663:i16)
              }
              frame "Z Position" {
              }
              frame "Save" {
                n336 = Build Array(w670) -> (w669:dbl[])
                n337 = call "Stage_position_ae.vi"("Position In"=w669, "StageID"="P541", "Enum"=enum16{"WRITE", "READ", "HOME", "SAVE HOME"}."SAVE HOME") -> ()  [unwired: 7 in, 2 out]
              }
              frame "Home" {
                n338 = call "Stage_position_ae.vi"("StageID"="P541", "Enum"=enum16{"WRITE", "READ", "HOME", "SAVE HOME"}."HOME") -> ("Position Out"=w674:dbl[])  [unwired: 8 in, 1 out]
                n339 = Index Array(array=w674, index=0) -> (element=w672:dbl)
                n340 = Multiply(x=w672, y=w676) -> (x*y=w678:dbl)
                n341 = Round To Nearest(number=w678) -> (nearest integer value=w679:dbl)
                n342 = To Word Integer(number=w679) -> (16bit integer=w677:i16)
              }
            }
            n343 = Bundle By Name(cluster=w639, "Z Axis Voltage (I16)"=w638) -> (w641:T21)
            n344 = call "Manual Controls Action Engine.vi"("Action"=enum16{"Read", "Write"}."Write", "Manual Controls In"=w641) -> ("Manual Controls Out"=w635:T21)  [unwired: 13 in]
            n345 = call "FPGA-7842R-Control V2.vi"("Action"=FPGA-7842R-Reference."Stage Control", "Manual Controls"=w635, "Initialize"=TRUE) -> ()  [unwired: 11 in, 2 out]
          }
          frame "Phase Comp Mirror - P841" {
            n346 = call "P841_Ctrl_Index.vi"("OldVal"=w694, "NewVal"=w693) -> ("Control out"=w691:refnum<vi>, "P841 Out"=w689:T8)  [unwired: 12 in]
            n347 = property class="Ctl"(reference=w691) -> ("Label.Text"=w690:string)  [unwired: 1 in, 2 out]
            n348 = Unbundle By Name(w689) -> ("Position (µm)"=w688:dbl, "Step Size (µm)"=w687:dbl)
            n349 = case shown="Default" w690 {
              tunnel: w688 -> [_ _ _ w707]
              tunnel: w687 -> [_ w700 w704 _]
              tunnel: [0.0 ("Position (µm)") w700 w703 w707] -> w683
              tunnel: [StageStates."MVR" ("Action") StageStates."MVR" ("Action") StageStates."MVR" ("Action") StageStates."MOVE" ("Action")] -> w686
              tunnel: [enum16{"MOVE", "MVR"}."MVR" ("MOVE/MVR") enum16{"MOVE", "MVR"}."MVR" ("MOVE/MVR") enum16{"MOVE", "MVR"}."MVR" ("MOVE/MVR") enum16{"MOVE", "MVR"}."MOVE" ("MOVE/MVR")] -> w685
              frame Default {
              }
              frame "Up P841" {
              }
              frame "Down P841" {
                n350 = Negate(x=w704) -> (-x=w703:dbl)
              }
              frame "Position (µm)" {
              }
            }
            n351 = Build Array(w683) -> (w682:dbl[])
          }
          frame "Sample Z Coarse - M227" {
            n352 = call "M227_Ctrl_Index.vi"("OldVal"=w723, "NewVal"=w722) -> ("Control Ref OUT"=w721:refnum<vi>, "M227 Out"=w719:T12)  [unwired: 12 in]
            n353 = property class="Ctl"(reference=w721) -> ("Label.Text"=w720:string)  [unwired: 1 in, 2 out]
            n354 = Unbundle By Name(w719) -> ("Step Size (mm)"=w718:dbl, "MM 1"=w711:dbl, "MM 2"=w710:dbl, "MM 3"=w709:dbl)
            n355 = case shown="\"MM 1\"" w720 {
              tunnel: w718 -> [_ _ _ _ w742 w747]
              tunnel: [bool[] [FALSE, FALSE, FALSE] bool[] [TRUE, TRUE, TRUE] bool[] [TRUE, TRUE, TRUE] bool[] [TRUE, TRUE, TRUE] bool[] [TRUE, TRUE, TRUE] bool[] [TRUE, TRUE, TRUE]] -> w716
              tunnel: [0.0 ("Step Size (mm)") w729 w733 w737 w742 w746] -> w713
              tunnel: [StageStates."POSITION" ("Action") StageStates."MOVE" ("Action") StageStates."MOVE" ("Action") StageStates."MOVE" ("Action") StageStates."MVR" ("Action") StageStates."MVR" ("Action")] -> w712
              tunnel: w711 -> [_ w729 _ _ _ _]
              tunnel: w710 -> [_ _ w733 _ _ _]
              tunnel: w709 -> [_ _ _ w737 _ _]
              tunnel: [enum16{"MOVE", "MVR"}."MVR" ("MOVE/MVR") enum16{"MOVE", "MVR"}."MOVE" ("MOVE/MVR") enum16{"MOVE", "MVR"}."MOVE" ("MOVE/MVR") enum16{"MOVE", "MVR"}."MOVE" ("MOVE/MVR") enum16{"MOVE", "MVR"}."MVR" ("MOVE/MVR") enum16{"MOVE", "MVR"}."MVR" ("MOVE/MVR")] -> w708
              frame Default {
              }
              frame "MM 1" {
              }
              frame "MM 2" {
              }
              frame "MM 3" {
              }
              frame "Up M227" {
              }
              frame "Down M227" {
                n356 = Negate(x=w747) -> (-x=w746:dbl)
              }
            }
            n357 = Build Array(w713, w713, w713) -> (w715:dbl[])
          }
          frame "Sample Stage XY - M686" {
            n358 = call "M686_Ctrl_Index.vi"("NewVal"=w762, "OldVal"=w763) -> ("M686 - out"=w760:T9, "Control out"=w761:refnum<vi>)  [unwired: 8 in]
            n359 = Unbundle By Name(w760) -> ("Step Size (um)"=w759:dbl, "X"=w758:dbl, "Y"=w757:dbl)
            n360 = property class="Ctl"(reference=w761) -> ("Label.Text"=w750:string)  [unwired: 1 in, 2 out]
            n361 = Unbundle By Name("Sample Stage XY - M686") -> ()  [unwired: 8 out]
            n362 = case shown="\"Left Button\"" w750 {
              tunnel: w759 -> [_ _ w775 w780 w788 w793 _]
              tunnel: w758 -> [_ _ _ _ _ _ w800]
              tunnel: w757 -> [_ _ _ _ _ _ w799]
              tunnel: [StageStates."POSITION" ("Action") StageStates."MOVE" ("Action") StageStates."MVR" ("Action") StageStates."MVR" ("Action") StageStates."MVR" ("Action") StageStates."MVR" ("Action") StageStates."MOVE" ("Action")] -> w755
              tunnel: [enum16{"MOVE", "MVR"}."MVR" ("MOVE/MVR") enum16{"MOVE", "MVR"}."MOVE" ("MOVE/MVR") enum16{"MOVE", "MVR"}."MVR" ("MOVE/MVR") enum16{"MOVE", "MVR"}."MVR" ("MOVE/MVR") enum16{"MOVE", "MVR"}."MVR" ("MOVE/MVR") enum16{"MOVE", "MVR"}."MVR" ("MOVE/MVR") enum16{"MOVE", "MVR"}."MOVE" ("MOVE/MVR")] -> w754
              tunnel: [w765 dbl[] [12.5, 12.5] w773 w781 w789 w795 w801] -> w752
              tunnel: [bool[] [FALSE, FALSE] bool[] [TRUE, TRUE] bool[] [TRUE, TRUE] bool[] [TRUE, TRUE] bool[] [TRUE, TRUE] bool[] [TRUE, TRUE] bool[] [TRUE, TRUE]] -> w751
              frame Default {
                w766 = 0.0 ("Step Size (mm)")
                n363 = Build Array(w766, w766) -> (w765:dbl[])
              }
              frame "Home Button" {
              }
              frame "Right Button" {
                n364 = Build Array(w775, 0.0 ("element")) -> (w773:dbl[])
              }
              frame "Left Button" {
                n365 = Negate(x=w780) -> (-x=w779:dbl)
                n366 = Build Array(w779, 0.0 ("element")) -> (w781:dbl[])
              }
              frame "Up Button" {
                n367 = Negate(x=w788) -> (-x=w787:dbl)
                n368 = Build Array(0.0 ("element"), w787) -> (w789:dbl[])
              }
              frame "Down Button" {
                n369 = Build Array(0.0 ("element"), w793) -> (w795:dbl[])
              }
              frame "X", "Y" {
                n370 = Build Array(w800, w799) -> (w801:dbl[])
              }
            }
          }
        }
        n371 = case shown="Default" w495 {
          frame Default {
          }
          frame "Upper Objective Z - N664" {
            n372 = while {
              i -> [w810]
              stop <- w806 stop-if-true
              n373 = call "Stage_position_ae.vi"("StageID"="N664", "Enum"=enum16{"WRITE", "READ", "HOME", "SAVE HOME"}."READ") -> ("Status Out"=w807:bool, "Position Out"=w817:dbl[])  [unwired: 8 in]
              n374 = Greater?(x=w810, y=200) -> (0:w809:bool)
              n375 = And(x=w807, y=w809) -> (x .and. y?=w806:bool)
              n376 = Wait (ms)(milliseconds to wait=u32 1) -> ()  [unwired: 1 out]
              n377 = Index Array(array=w817, index=0) -> (element=w816:dbl)
              n378 = Select(t=u32 16777215, s=w806, f=u32 6618880) -> (s? t:f=w811:u32)
              n379 = property on="Position (mm)" class="DigNum (strict)"("Value"=w816, "NumText.BG Color"=w811) -> ()  [unwired: 2 in, 2 out]
            }
          }
          frame "Cavity Translation Z - ASI" {
            n380 = while {
              shift-right: [w824] -> _
              shift-left: TRUE ("Status Out") -> [w829]
              stop <- w828 stop-if-true
              n381 = call "Stage_position_ae.vi"("StageID"="ASI", "Enum"=enum16{"WRITE", "READ", "HOME", "SAVE HOME"}."READ") -> ("Status Out"=w824:bool, "Position Out"=w832:dbl[])  [unwired: 8 in]
              n382 = Greater?(x=w824, y=w829) -> (0:w828:bool)
              n383 = Wait (ms)(milliseconds to wait=u32 1) -> ()  [unwired: 1 out]
              n384 = Index Array(array=w832, index=0) -> (element=w822:dbl)
              n385 = Divide(x=w822, y=10.0) -> (x/y=w823:dbl)
              n386 = Select(t=u32 16777215, s=w824, f=u32 6618880) -> (s? t:f=w825:u32)
              n387 = property on="Z (um)" class="DigNum (strict)"("Value"=w823, "NumText.BG Color"=w825) -> ()  [unwired: 2 in, 2 out]
            }
          }
        }
        n388 = control-ref of="Abort AllStage"() -> (w486:refnum<vi>)
        n389 = call "AllStage_Limits_Array.vi"("Step(um)/Position(units)"=w493, "Axis"=w492, "Stage ID"=w494, "MOVE/MVR"=w491) -> ("Positions"=w489:dbl[], "Boolean Array"=w488:bool[], "Stage ID"=w490:string)  [unwired: 4 in, 1 out]
        n390 = call "AE_AllStages_Action V2.vi"("Velocity"=w487, "Abort"=w486, "Positions"=w489, "Axis"=w488, "Stage ID"=w490, "Action"=w485) -> ()  [unwired: 3 in, 3 out]
      }
      event "Stages": Value Change {
        n391 = event-data() -> ("NewVal"=w846:T11)  [unwired: 1 in, 2 out]
        n392 = Unbundle By Name(w846) -> ("M686"=w834:bool, "P841"=w844:bool, "ASI"=w842:bool, "N664"=w840:bool, "P612"=w838:bool, "M227"=w836:bool)
        n393 = call "All_Stages_Aloha.vi"("Aloha"=w834, "Stage ID"="M686") -> ()  [unwired: 9 in, 1 out]
        n394 = call "All_Stages_Aloha.vi"("Aloha"=w844, "Stage ID"="P841") -> ()  [unwired: 9 in, 1 out]
        n395 = call "All_Stages_Aloha.vi"("Aloha"=w842, "Stage ID"="ASI") -> ()  [unwired: 9 in, 1 out]
        n396 = call "All_Stages_Aloha.vi"("Aloha"=w840, "Stage ID"="N664") -> ()  [unwired: 9 in, 1 out]
        n397 = call "All_Stages_Aloha.vi"("Aloha"=w838, "Stage ID"="P612") -> ()  [unwired: 9 in, 1 out]
        n398 = call "All_Stages_Aloha.vi"("Aloha"=w836, "Stage ID"="M227") -> ()  [unwired: 9 in, 1 out]
      }
      event Value Change {
        n399 = event-data() -> ("CtlRef"=w850:refnum<vi>, "NewVal"=w847:T14)  [unwired: 1 in, 1 out]
        n400 = property class="Bool (strict)"(reference=w850) -> ("Label.Text"=w849:string)  [unwired: 1 in, 2 out]
        n401 = case shown="\"Focus Lock\"" w849 {
          tunnel: w847 -> [w851 w865 w879 w883 w897 w910 w927]
          frame "SLM", Default {
            n402 = case shown="True" w851 {
              frame False {
                n403 = To Variant(anything=TRUE) -> (Variant=w857:variant)
                n404 = call "SLM AE.vi"("Action"=enum16{"READ", "WRITE"}."READ") -> ("SLM Ref Out"=w858:refnum<vi>)  [unwired: 10 in]
                n405 = invoke class="VI" method="Ctrl Val.Set"(reference=w858, "Control Name"="Exit", "Value"=w857) -> (reference out=w854:refnum<vi>, error out=w853:errorcluster)  [unwired: 2 in, 3 out]
                n406 = invoke on="Hamamatsu LCOS" class="SubPnl" method="Remove VI"(error in=w853) -> (error out=w852:errorcluster)  [unwired: 2 in, 2 out]
                n407 = Close Reference(reference=w854, error in (no error)=w852) -> ()  [unwired: 1 out]
              }
              frame True {
                n408 = Open VI Reference(vi path=path "C:/Users/ED STED/Documents/Test Control Software/Host VIs/SLM_V2/SLM Control.vi") -> (vi reference=w863:refnum<vi>)  [unwired: 5 in, 1 out]
                n409 = invoke class="VI" method="Run VI"(reference=w863, "Wait until done"=FALSE ("Wait Until Done")) -> (reference out=w860:refnum<vi>)  [unwired: 3 in, 4 out]
                n410 = invoke on="Hamamatsu LCOS" class="SubPanel" method="Insert VI"("VI Ref"=w860) -> ()  [unwired: 3 in, 4 out]
                n411 = call "SLM AE.vi"("Action"=enum16{"READ", "WRITE"}."WRITE", "SLM Ref In"=w860) -> ()  [unwired: 9 in, 1 out]
              }
            }
          }
          frame "DM" {
            n412 = case shown="True" w865 {
              frame False {
                n413 = call "DM_Ref_AE.vi"("Action"=enum16{"READ", "WRITE"}."READ") -> ("DM Ref Out"=w872:refnum<vi>)  [unwired: 10 in]
                n414 = To Variant(anything=TRUE) -> (Variant=w871:variant)
                n415 = invoke class="VI" method="Ctrl Val.Set"(reference=w872, "Control Name"="Exit", "Value"=w871) -> (reference out=w868:refnum<vi>, error out=w867:errorcluster)  [unwired: 2 in, 3 out]
                n416 = invoke on="BM Multi" class="SubPnl" method="Remove VI"(error in=w867) -> (error out=w866:errorcluster)  [unwired: 2 in, 2 out]
                n417 = Close Reference(reference=w868, error in (no error)=w866) -> ()  [unwired: 1 out]
              }
              frame True {
                n418 = Open VI Reference(vi path=path "C:/Users/ED STED/Documents/Test Control Software/Host VIs/DM_Dual_V2/Dual_DM_Control_Main_V6.vi") -> (vi reference=w877:refnum<vi>)  [unwired: 5 in, 1 out]
                n419 = invoke class="VI" method="Run VI"(reference=w877, "Wait until done"=FALSE ("Wait Until Done")) -> (reference out=w874:refnum<vi>)  [unwired: 3 in, 4 out]
                n420 = invoke on="BM Multi" class="SubPanel" method="Insert VI"("VI Ref"=w874) -> ()  [unwired: 3 in, 4 out]
                n421 = call "DM_Ref_AE.vi"("Action"=enum16{"READ", "WRITE"}."WRITE", "DM Ref In"=w874) -> ()  [unwired: 9 in, 1 out]
              }
            }
          }
          frame "Sequence" {
            n422 = case shown="False" w879 {
              tunnel: [T25."Disabled and Grayed Out" ("Disabled") T25."Enabled" ("Disabled")] -> w880
              frame False {
              }
              frame True {
              }
            }
            n423 = property on="Sequence Cluster" class="Clust"("DisabledEnum"=w880) -> ()  [unwired: 2 in, 2 out]
          }
          frame "Timing" {
            n424 = case shown="True" w883 {
              frame False {
                n425 = To Variant(anything=TRUE) -> (Variant=w888:variant)
                n426 = call "GateDelay AE.vi"("Action"=enum16{"READ", "WRITE"}."READ") -> ("Gate Delay Ref Out"=w889:refnum<vi>)  [unwired: 10 in]
                n427 = invoke class="VI" method="Ctrl Val.Set"(reference=w889, "Control Name"="Exit", "Value"=w888) -> (reference out=w884:refnum<vi>, error out=w885:errorcluster)  [unwired: 2 in, 3 out]
                n428 = invoke on="Timing" class="SubPnl" method="Remove VI"(error in=w885) -> (error out=w891:errorcluster)  [unwired: 2 in, 2 out]
                n429 = Close Reference(reference=w884, error in (no error)=w891) -> ()  [unwired: 1 out]
              }
              frame True {
                n430 = Open VI Reference(vi path=path "C:/Users/ED STED/Documents/Test Control Software/Host VIs/Time Delay/GateDelay_Control_V3.vi") -> (vi reference=w894:refnum<vi>)  [unwired: 5 in, 1 out]
                n431 = invoke class="VI" method="Run VI"(reference=w894, "Wait until done"=FALSE ("Wait Until Done")) -> (reference out=w893:refnum<vi>)  [unwired: 3 in, 4 out]
                n432 = invoke on="Timing" class="SubPanel" method="Insert VI"("VI Ref"=w893) -> ()  [unwired: 3 in, 4 out]
                n433 = call "GateDelay AE.vi"("Action"=enum16{"READ", "WRITE"}."WRITE", "Gate Delay Ref In"=w893) -> ()  [unwired: 9 in, 1 out]
              }
            }
          }
          frame "Camera" {
            n434 = case shown="False" w897 {
              frame False {
                n435 = To Variant(anything=TRUE) -> (Variant=w898:variant)
                n436 = call "Camera_Ref_HX.vi"("Action"=enum16{"READ", "WRITE"}."READ") -> ("Alignment Ref Out"=w902:refnum<vi>)  [unwired: 10 in]
                n437 = invoke class="VI" method="Ctrl Val.Set"(reference=w902, "Control Name"="Exit", "Value"=w898) -> (reference out=w901:refnum<vi>)  [unwired: 2 in, 4 out]
                n438 = invoke on="Tool Box" class="SubPnl" method="Remove VI"() -> (error out=w903:errorcluster)  [unwired: 3 in, 2 out]
                n439 = Close Reference(reference=w901, error in (no error)=w903) -> ()  [unwired: 1 out]
              }
              frame True {
                n440 = Open VI Reference(vi path=path "C:/Users/ED STED/Documents/Test Control Software/Host VIs/Camera/uEye_Control_V1.vi") -> (vi reference=w907:refnum<vi>)  [unwired: 5 in, 1 out]
                n441 = invoke class="VI" method="Run VI"(reference=w907, "Wait until done"=FALSE ("Wait Until Done")) -> (reference out=w906:refnum<vi>)  [unwired: 3 in, 4 out]
                n442 = invoke on="Tool Box" class="SubPnl" method="Insert VI"("VI Ref"=w906) -> ()  [unwired: 3 in, 4 out]
                n443 = call "Camera_Ref_HX.vi"("Action"=enum16{"READ", "WRITE"}."WRITE", "Alignment Ref In"=w906) -> ()  [unwired: 9 in, 1 out]
              }
            }
          }
          frame "Focus Lock" {
            n444 = case shown="True" w910 {
              frame False {
                n445 = call "Lock Control AE.vi"("Action"=Standard_Action_for_Focus_Lock."Read") -> ("Lock Control  out"=w913:T42)  [unwired: 1 in]
                n446 = Bundle By Name(cluster=w913, "EXIT"=TRUE) -> (w911:T42)
                n447 = call "FocusLock_Ref_HX.vi"("Action"=enum16{"READ", "WRITE"}."READ") -> ("FocusLock Ref Out"=w919:refnum<vi>)  [unwired: 10 in]
                n448 = To Variant(anything=w911) -> (Variant=w917:variant)
                n449 = invoke class="VI" method="Ctrl Val.Set"(reference=w919, "Control Name"="Lock Control", "Value"=w917) -> (reference out=w918:refnum<vi>, error out=w916:errorcluster)  [unwired: 2 in, 3 out]
                n450 = invoke on="Focus Lock\nFocus Lock Panel" class="SubPnl" method="Remove VI"(error in=w916) -> (error out=w920:errorcluster)  [unwired: 2 in, 2 out]
                n451 = Close Reference(reference=w918, error in (no error)=w920) -> ()  [unwired: 1 out]
              }
              frame True {
                n452 = Open VI Reference(vi path=path "C:/Users/ED STED/Documents/Test Control Software/Host VIs/Focus Lock/FocusLock Control v3.vi") -> (vi reference=w924:refnum<vi>)  [unwired: 5 in, 1 out]
                n453 = invoke class="VI" method="Run VI"(reference=w924, "Wait until done"=FALSE ("Wait Until Done")) -> (reference out=w923:refnum<vi>)  [unwired: 3 in, 4 out]
                n454 = invoke on="Focus Lock\nFocus Lock Panel" class="SubPnl" method="Insert VI"("VI Ref"=w923) -> ()  [unwired: 3 in, 4 out]
                n455 = call "FocusLock_Ref_HX.vi"("Action"=enum16{"READ", "WRITE"}."WRITE", "FocusLock Ref In"=w923) -> ()  [unwired: 9 in, 1 out]
              }
            }
          }
          frame "Stage Monitor" {
            n456 = case shown="True" w927 {
              frame False {
                n457 = call "StageMonitor_Ref_HX.vi"("Action"=enum16{"READ", "WRITE"}."READ") -> ("StageMonitor Ref Out"=w930:refnum<vi>)  [unwired: 10 in]
                n458 = To Variant(anything=TRUE) -> (Variant=w933:variant)
                n459 = invoke class="VI" method="Ctrl Val.Set"(reference=w930, "Control Name"="Exit", "Value"=w933) -> (reference out=w934:refnum<vi>, error out=w932:errorcluster)  [unwired: 2 in, 3 out]
                n460 = invoke on="Tool Box 2" class="SubPnl" method="Remove VI"(error in=w932) -> (error out=w935:errorcluster)  [unwired: 2 in, 2 out]
                n461 = Close Reference(reference=w934, error in (no error)=w935) -> ()  [unwired: 1 out]
              }
              frame True {
                n462 = Open VI Reference(vi path=path "C:/Users/ED STED/Documents/Test Control Software/Host VIs/Stages/Stage Monitor/Stage Monitor.vi") -> (vi reference=w938:refnum<vi>)  [unwired: 5 in, 1 out]
                n463 = invoke class="VI" method="Run VI"(reference=w938, "Wait until done"=FALSE ("Wait Until Done")) -> (reference out=w937:refnum<vi>)  [unwired: 3 in, 4 out]
                n464 = invoke on="Tool Box 2" class="SubPnl" method="Insert VI"("VI Ref"=w937) -> ()  [unwired: 3 in, 4 out]
                n465 = call "StageMonitor_Ref_HX.vi"("Action"=enum16{"READ", "WRITE"}."WRITE", "StageMonitor Ref In"=w937) -> ()  [unwired: 9 in, 1 out]
              }
            }
          }
        }
      }
      event Value Change {
        n466 = event-data() -> ("CtlRef"=w946:refnum<vi>, "OldVal"=w944:variant, "NewVal"=w943:variant)  [unwired: 1 in]
        n467 = property class="Clust"(reference=w946) -> ("Label.Text"=w945:string)  [unwired: 1 in, 2 out]
        n468 = call "Graph Ref AE.vi"("Action"=enum16{"READ", "WRITE"}."READ") -> ("Graph Ref Out"=w941:refnum<vi>[])  [unwired: 10 in]
        n469 = case shown="\"Graph Tools\"" w945 {
          tunnel: w944 -> [_ w953 w1009]
          tunnel: w943 -> [_ w954 w1008]
          tunnel: w941 -> [_ w948 w1001]
          frame Default {
          }
          frame "Display Controls" {
            n470 = call "Display_Controls_Ctrl_Index.vi"("OldVal"=w953, "NewVal"=w954) -> ("Control Ref OUT"=w952:refnum<vi>, "Display Controls Out"=w950:T3)  [unwired: 12 in]
            n471 = property class="Ctl"(reference=w952) -> ("Label.Text"=w951:string)  [unwired: 1 in, 2 out]
            n472 = Unbundle By Name(w950) -> ("Single Screen"=w949:bool)
            n473 = case shown="\"Single Screen\", Default" w951 {
              tunnel: w949 -> [w962 _ _]
              tunnel: w948 -> [_ w987 w994]
              frame "Single Screen", Default {
                n474 = property class="App"() -> ("Disp.AllMonitors"=w961:T43)  [unwired: 2 in, 2 out]
                n475 = Index Array(array=w961, index #1=2 ("index"), index #2=0 ("index")) -> (element #1=w958:T44, element #2=w957:T44)
                n476 = control-ref of="This VI"() -> (w956:refnum<vi>)
                n477 = case shown="False" w962 {
                  tunnel: w958 -> [w966 _]
                  tunnel: w957 -> [w965 w977]
                  tunnel: w956 -> [w964 w975]
                  tunnel: T28 {"Left"=0, "Top"=0, "Right"=0, "Bottom"=0} ("Front Panel Window:Window Bounds") -> [w963 w976]
                  frame False {
                    w971 = i16 0
                    n478 = Unbundle By Name(w965) -> ("Bounds.Left"=w968:i16, "Bounds.Bottom"=w969:i16, "Bounds.Top"=w970:i16)
                    n479 = Unbundle By Name(w966) -> ("Bounds.Right"=w967:i16)
                    n480 = Subtract(x=w967, y=w968) -> (x-y=w972:i16)
                    n481 = Subtract(x=w969, y=w970) -> (x-y=w973:i16)
                    n482 = Bundle By Name(cluster=w963, "Left"=w971, "Top"=w971, "Right"=w972, "Bottom"=w973) -> (w974:T28)
                    n483 = property class="VI"(reference=w964, "Front Panel.WinBounds"=w974) -> ()  [unwired: 1 in, 2 out]
                  }
                  frame True {
                    w980 = i16 0
                    n484 = Unbundle By Name(w977) -> ("Bounds.Right"=w983:i16, "Bounds.Bottom"=w982:i16, "Bounds.Top"=w981:i16)
                    n485 = Subtract(x=w982, y=w981) -> (x-y=w979:i16)
                    n486 = Bundle By Name(cluster=w976, "Left"=w980, "Top"=w980, "Right"=w983, "Bottom"=w979) -> (w978:T28)
                    n487 = property class="VI"(reference=w975, "Front Panel.WinBounds"=w978) -> (reference out=w985:refnum<vi>)  [unwired: 1 in, 1 out]
                    n488 = property class="VI"(reference=w985, "FP.State"=T29."Maximized" ("Front Panel Window:State")) -> ()  [unwired: 1 in, 2 out]
                  }
                }
              }
              frame "Add Display" {
                w988 = u16 0 items=["Read", "Write"] ("Action")
                w992 = u16 1 items=["Read", "Write"] ("Action")
                n489 = property on="Add Display" class="Bool (strict)"("Value"=FALSE) -> ()  [unwired: 2 in, 2 out]
                n490 = call "Arange_Displays_V2.vi"("Action"=w988) -> ("Number of Channels OUT"=w989:i32)  [unwired: 14 in]
                n491 = Increment(x=w989) -> (x+1=w991:i32)
                n492 = call "Arange_Displays_V2.vi"("Display References"=w987, "Action"=w992, "Number of Channels"=w991, "Aspect Ratio (h/w)"=1.0) -> ()  [unwired: 11 in, 1 out]
              }
              frame "Remove Display" {
                w995 = u16 0 items=["Read", "Write"] ("Action")
                w999 = u16 1 items=["Read", "Write"] ("Action")
                n493 = call "Arange_Displays_V2.vi"("Action"=w995) -> ("Number of Channels OUT"=w996:i32)  [unwired: 14 in]
                n494 = Decrement(x=w996) -> (x-1=w998:i32)
                n495 = call "Arange_Displays_V2.vi"("Display References"=w994, "Action"=w999, "Number of Channels"=w998, "Aspect Ratio (h/w)"=1.0) -> ()  [unwired: 11 in, 1 out]
                n496 = property on="Remove Display" class="Bool (strict)"("Value"=FALSE) -> ()  [unwired: 2 in, 2 out]
              }
            }
          }
          frame "Graph Tools" {
            n497 = call "Graph_Controls_Ctrl_Index.vi"("OldVal"=w1009, "NewVal"=w1008) -> ("Control Ref OUT"=w1007:refnum<vi>, "Graph Tools Out"=w1006:T4)  [unwired: 12 in]
            n498 = property class="Ctl"(reference=w1007) -> (reference out=w1003:refnum<vi>, "Label.Text"=w1002:string)  [unwired: 1 in, 1 out]
            n499 = Unbundle By Name(w1006) -> ("Show Cursor"=w1005:bool, "Auto Scale"=w1004:bool, "Color Map"=w1000:T45)
            n500 = case shown="\"Load File\"" w1002 {
              selector: w1002 -> [_ _ _ w1080 _ _ _ _]
              tunnel: w1005 -> [_ w1049 _ _ _ _ _ _]
              tunnel: w1004 -> [_ _ w1069 _ _ _ _ _]
              tunnel: w1001 -> [w1018 w1048 w1070 w1073 w1110 w1128 w1141 w1149]
              tunnel: w1003 -> [_ _ _ _ _ _ _ _]
              tunnel: w1002 -> [_ _ _ w1075 _ _ _ _]
              tunnel: w1000 -> [w1021 _ _ _ _ _ _ _]
              frame "Apply Color" {
                n501 = control-ref of="This VI"() -> (w1020:refnum<vi>)
                n502 = call "GetDisplayClick.vi"("Display REFs In"=w1018, "Calling VI REF"=w1020) -> ("Display Index"=w1019:i32)  [unwired: 13 in]
                n503 = Index Array(array=w1018, index=w1019) -> (element=w1017:refnum<vi>)
                n504 = property class="IntGraph (strict)"(reference=w1017) -> (reference out=w1013:refnum<vi>, error out=w1010:errorcluster, "ZScale.Maximum"=w1016:dbl)  [unwired: 1 in]
                n505 = case shown="\"Gray\"" w1021 {
                  tunnel: [cluster{dbl, u32}[] [{0.0, 0}, {0.07843137254901933, 131072}, {0.15686274509805287, 196608}, {0.235294117647058, 327680}, {0.3137254901960773, 458752}, {0.39215686274509665, 589824}, {0.47058823529410176, 720896}, {0.5490196078431353, 851971}, {0.6274509803921546, 983043}, {0.705882352941174, 1114115}, {0.7843137254902075, 1245187}, {0.8627450980392268, 1376259}, {0.941176470588232, 1507331}, {1.0196078431372513, 1638403}, {1.0980392156862848, 1769475}, {1.1764705882353041, 1769479}, {1.2549019607843093, 2031623}, {1.3333333333333286, 2162695}, {1.4117647058823621, 2293767}, {1.4901960784313673, 2424839}, {1.5686274509803866, 2555911}, {1.647058823529406, 2686983}, {1.7254901960784395, 2818055}, {1.8039215686274588, 2949127}, {1.882352941176464, 3080203}, {1.9607843137254832, 3211275}, {2.0392156862745168, 3342347}, {2.117647058823522, 3473419}, {2.1960784313725554, 3604491}, {2.2745098039215605, 3735563}, {2.352941176470594, 3866635}, {2.431372549019599, 3867403}, {2.5098039215686327, 4129547}, {2.588235294117638, 4260619}, {2.6666666666666714, 4391691}, {2.7450980392156907, 4522763}, {2.823529411764696, 4653839}, {2.901960784313715, 4784911}, {2.9803921568627487, 4915983}, {3.058823529411768, 5178127}, {3.1372549019607874, 5309199}, {3.2156862745097925, 5440271}, {3.294117647058826, 5571343}, {3.3725490196078454, 5702415}, {3.4509803921568647, 5703439}, {3.52941176470587, 5965583}, {3.6078431372549034, 6096655}, {3.6862745098039227, 6227727}, {3.764705882352942, 6358799}, {3.8431372549019756, 6489871}, {3.9215686274509807, 6620943}, {4.0, 6752015}, {4.078431372549019, 6883087}, {4.1568627450980244, 7015183}, {4.235294117647058, 7146255}, {4.313725490196077, 7277327}, {4.392156862745097, 7408399}, {4.470588235294102, 7539471}, {4.549019607843135, 7670543}, {4.627450980392155, 7801615}, {4.705882352941174, 8063759}, {4.784313725490179, 8194831}, {4.862745098039213, 8326927}, {4.941176470588232, 8457999}, {5.019607843137251, 8589075}, {5.098039215686285, 8720147}, {5.17647058823529, 8851219}, {5.254901960784309, 8982291}, {5.333333333333329, 9113363}, {5.411764705882362, 9114387}, {5.490196078431367, 9376531}, {5.568627450980401, 9507603}, {5.647058823529406, 9638675}, {5.7254901960784395, 9769747}, {5.803921568627445, 9901843}, {5.882352941176478, 10032915}, {5.960784313725483, 10163987}, {6.039215686274517, 10229523}, {6.117647058823522, 10295059}, {6.196078431372555, 10427155}, {6.2745098039215605, 10558227}, {6.352941176470594, 10689299}, {6.431372549019599, 10820371}, {6.509803921568633, 10886931}, {6.588235294117638, 10952467}, {6.666666666666671, 11083539}, {6.745098039215691, 11214611}, {6.82352941176471, 11215635}, {6.901960784313715, 11477779}, {6.980392156862749, 11543315}, {7.058823529411768, 11608851}, {7.137254901960787, 11740947}, {7.215686274509821, 11806483}, {7.294117647058826, 11872019}, {7.372549019607845, 12004115}, {7.450980392156865, 12135187}, {7.529411764705898, 12266259}, {7.607843137254903, 12267283}, {7.686274509803923, 12398355}, {7.764705882352942, 12529427}, {7.843137254901947, 12530451}, {7.921568627450981, 12595987}, {8.0, 12530451}, {8.07843137254902, 12793619}, {8.156862745098024, 12794131}, {8.235294117647058, 12794643}, {8.313725490196077, 13056787}, {8.392156862745097, 13057299}, {8.47058823529413, 13057811}, {8.549019607843135, 13188883}, {8.627450980392155, 13320979}, {8.705882352941174, 13386515}, {8.784313725490179, 13452563}, {8.862745098039213, 13584147}, {8.941176470588232, 13584659}, {9.019607843137251, 13585171}, {9.098039215686256, 13585683}, {9.17647058823529, 13717267}, {9.254901960784323, 13848339}, {9.333333333333329, 13849363}, {9.411764705882362, 13849875}, {9.490196078431367, 13850387}, {9.5686274509804, 13981459}, {9.647058823529406, 14113555}, {9.72549019607844, 14114067}, {9.803921568627445, 14114579}, {9.882352941176478, 14115091}, {9.960784313725483, 14246675}, {10.039215686274517, 14377747}, {10.117647058823522, 14378771}, {10.196078431372555, 14379283}, {10.27450980392156, 14379539}, {10.352941176470594, 14379795}, {10.4313725490196, 14380819}, {10.509803921568633, 14511891}, {10.588235294117638, 14643987}, {10.666666666666671, 14644503}, {10.745098039215677, 14645015}, {10.82352941176471, 14645527}, {10.901960784313744, 14646039}, {10.980392156862749, 14646551}, {11.058823529411768, 14778135}, {11.137254901960787, 14909207}, {11.215686274509821, 14910231}, {11.294117647058826, 14910747}, {11.372549019607845, 14911259}, {11.450980392156865, 14911771}, {11.52941176470587, 14912283}, {11.607843137254903, 14912797}, {11.686274509803923, 15044383}, {11.764705882352942, 15175455}, {11.843137254901947, 15175967}, {11.92156862745098, 15176479}, {12.0, 15176991}, {12.07843137254902, 15177507}, {12.156862745098053, 15178019}, {12.235294117647058, 15178531}, {12.313725490196092, 15310115}, {12.392156862745097, 15441701}, {12.47058823529413, 15441959}, {12.549019607843135, 15442215}, {12.627450980392155, 15442727}, {12.705882352941174, 15443243}, {12.784313725490179, 15443755}, {12.862745098039213, 15444269}, {12.941176470588246, 15444783}, {13.019607843137251, 15444783}, {13.098039215686285, 15576367}, {13.17647058823529, 15707953}, {13.25490196078431, 15708467}, {13.333333333333329, 15708979}, {13.411764705882362, 15708981}, {13.490196078431367, 15708983}, {13.568627450980387, 15710011}, {13.647058823529406, 15710523}, {13.725490196078411, 15711037}, {13.803921568627459, 15711039}, {13.882352941176464, 15711553}, {13.960784313725512, 15843139}, {14.039215686274517, 15974213}, {14.117647058823522, 15974215}, {14.196078431372541, 15974217}, {14.27450980392156, 15974219}, {14.352941176470594, 15975755}, {14.431372549019613, 15976271}, {14.509803921568633, 15976785}, {14.588235294117666, 15977299}, {14.666666666666671, 15977301}, {14.745098039215677, 15977815}, {14.82352941176471, 15978327}, {14.901960784313744, 15978331}, {14.980392156862749, 16109917}, {15.058823529411768, 16241503}, {15.137254901960787, 16241505}, {15.215686274509792, 16242019}, {15.294117647058826, 16242535}, {15.372549019607845, 16242537}, {15.450980392156865, 16242539}, {15.529411764705898, 16243563}, {15.607843137254903, 16243567}, {15.686274509803908, 16244081}, {15.764705882352942, 16244595}, {15.843137254901947, 16244599}, {15.92156862745098, 16244601}, {16.0, 16244603}, {16.07843137254902, 16245627}, {16.156862745098024, 16245631}, {16.235294117647058, 16245633}, {16.313725490196077, 16246147}, {16.392156862745097, 16246663}, {16.47058823529413, 16377735}, {16.549019607843135, 16508811}, {16.62745098039217, 16508815}, {16.705882352941174, 16509839}, {16.78431372549018, 16509843}, {16.862745098039213, 16509845}, {16.941176470588232, 16509847}, {17.01960784313725, 16510361}, {17.098039215686256, 16510875}, {17.17647058823529, 16510879}, {17.25490196078431, 16510881}, {17.33333333333333, 16510883}, {17.411764705882362, 16511399}, {17.49019607843138, 16511911}, {17.568627450980387, 16511915}, {17.647058823529406, 16511917}, {17.72549019607844, 16511919}, {17.80392156862746, 16511923}, {17.882352941176464, 16512437}, {17.960784313725483, 16512951}, {18.03921568627449, 16512955}, {18.117647058823522, 16512957}, {18.19607843137254, 16512959}, {18.27450980392156, 16512961}, {18.352941176470594, 16512963}, {18.431372549019613, 16512967}, {18.509803921568633, 16513481}, {18.588235294117638, 16513995}, {18.66666666666667, 16513999}, {18.74509803921569, 16514001}, {18.82352941176471, 16514003}, {18.901960784313744, 16514005}, {18.98039215686275, 16514007}, {19.058823529411754, 16514011}, {19.137254901960787, 16514013}, {19.215686274509792, 16514015}, {19.294117647058826, 16514019}, {19.372549019607845, 16514021}, {19.450980392156865, 16514023}, {19.52941176470587, 16514027}, {19.607843137254918, 16514029}, {19.686274509803923, 16514031}, {19.764705882352942, 16514035}, {19.843137254901947, 16514037}, {19.921568627450995, 16514039}, {20.0, 16514043}] ("Z Scale.Marker Values[]") cluster{dbl, u32}[] [{0.0, 0}, {85.0, 16711680}, {108.0, 16729344}, {127.0, 16744192}, {132.0, 16747520}, {140.0, 16753920}, {157.0, 16766720}, {170.0, 16776960}, {245.0, 16777184}, {250.0, 16777200}, {255.0, 16777215}] ("Z Scale.Marker Values[]") cluster{dbl, u32}[] [{0.0, 0}, {255.0, 16777215}] ("Z Scale.Marker Values[]") cluster{dbl, u32}[] [{0.0, 0}, {255.0, 16711680}] ("Z Scale.Marker Values[]") cluster{dbl, u32}[] [{0.0, 0}, {255.0, 65280}] ("Z Scale.Marker Values[]") cluster{dbl, u32}[] [{0.0, 0}, {255.0, 255}] ("Z Scale.Marker Values[]") cluster{dbl, u32}[] [{0.0, 0}, {255.0, 65535}] ("Z Scale.Marker Values[]") cluster{dbl, u32}[] [{0.0, 0}, {255.0, 16711935}] ("Z Scale.Marker Values[]") cluster{dbl, u32}[] [{0.0, 0}, {255.0, 16776960}] ("Z Scale.Marker Values[]") cluster{dbl, u32}[] [{0.0, 0}, {170.0, 16711680}, {245.0, 16777184}, {250.0, 16777200}, {255.0, 16448250}] ("Z Scale.Marker Values[]") cluster{dbl, u32}[] [{0.0, 0}, {170.0, 65280}, {245.0, 16777184}, {250.0, 16777200}, {255.0, 16448250}] ("Z Scale.Marker Values[]") cluster{dbl, u32}[] [{0.0, 0}, {170.0, 255}, {245.0, 16777184}, {250.0, 16777200}, {255.0, 16448250}] ("Z Scale.Marker Values[]") cluster{dbl, u32}[] [{0.0, 0}, {1.0, 131072}, {2.0, 196608}, {3.0, 327680}, {4.0, 458752}, {5.0, 589824}, {6.0, 720896}, {7.0, 851971}, {8.0, 983043}, {9.0, 1114115}, {10.0, 1245187}, {11.0, 1376259}, {12.0, 1507331}, {13.0, 1638403}, {14.0, 1769475}, {15.0, 1769479}, {16.0, 2031623}, {17.0, 2162695}, {18.0, 2293767}, {19.0, 2424839}, {20.0, 2555911}, {21.0, 2686983}, {22.0, 2818055}, {23.0, 2949127}, {24.0, 3080203}, {25.0, 3211275}, {26.0, 3342347}, {27.0, 3473419}, {28.0, 3604491}, {29.0, 3735563}, {30.0, 3866635}, {31.0, 3867403}, {32.0, 4129547}, {33.0, 4260619}, {34.0, 4391691}, {35.0, 4522763}, {36.0, 4653839}, {37.0, 4784911}, {38.0, 4915983}, {39.0, 5178127}, {40.0, 5309199}, {41.0, 5440271}, {42.0, 5571343}, {43.0, 5702415}, {44.0, 5703439}, {45.0, 5965583}, {46.0, 6096655}, {47.0, 6227727}, {48.0, 6358799}, {49.0, 6489871}, {50.0, 6620943}, {51.0, 6752015}, {52.0, 6883087}, {53.0, 7015183}, {54.0, 7146255}, {55.0, 7277327}, {56.0, 7408399}, {57.0, 7539471}, {58.0, 7670543}, {59.0, 7801615}, {60.0, 8063759}, {61.0, 8194831}, {62.0, 8326927}, {63.0, 8457999}, {64.0, 8589075}, {65.0, 8720147}, {66.0, 8851219}, {67.0, 8982291}, {68.0, 9113363}, {69.0, 9114387}, {70.0, 9376531}, {71.0, 9507603}, {72.0, 9638675}, {73.0, 9769747}, {74.0, 9901843}, {75.0, 10032915}, {76.0, 10163987}, {77.0, 10229523}, {78.0, 10295059}, {79.0, 10427155}, {80.0, 10558227}, {81.0, 10689299}, {82.0, 10820371}, {83.0, 10886931}, {84.0, 10952467}, {85.0, 11083539}, {86.0, 11214611}, {87.0, 11215635}, {88.0, 11477779}, {89.0, 11543315}, {90.0, 11608851}, {91.0, 11740947}, {92.0, 11806483}, {93.0, 11872019}, {94.0, 12004115}, {95.0, 12135187}, {96.0, 12266259}, {97.0, 12267283}, {98.0, 12398355}, {99.0, 12529427}, {100.0, 12530451}, {101.0, 12595987}, {102.0, 12530451}, {103.0, 12793619}, {104.0, 12794131}, {105.0, 12794643}, {106.0, 13056787}, {107.0, 13057299}, {108.0, 13057811}, {109.0, 13188883}, {110.0, 13320979}, {111.0, 13386515}, {112.0, 13452563}, {113.0, 13584147}, {114.0, 13584659}, {115.0, 13585171}, {116.0, 13585683}, {117.0, 13717267}, {118.0, 13848339}, {119.0, 13849363}, {120.0, 13849875}, {121.0, 13850387}, {122.0, 13981459}, {123.0, 14113555}, {124.0, 14114067}, {125.0, 14114579}, {126.0, 14115091}, {127.0, 14246675}, {128.0, 14377747}, {129.0, 14378771}, {130.0, 14379283}, {131.0, 14379539}, {132.0, 14379795}, {133.0, 14380819}, {134.0, 14511891}, {135.0, 14643987}, {136.0, 14644503}, {137.0, 14645015}, {138.0, 14645527}, {139.0, 14646039}, {140.0, 14646551}, {141.0, 14778135}, {142.0, 14909207}, {143.0, 14910231}, {144.0, 14910747}, {145.0, 14911259}, {146.0, 14911771}, {147.0, 14912283}, {148.0, 14912797}, {149.0, 15044383}, {150.0, 15175455}, {151.0, 15175967}, {152.0, 15176479}, {153.0, 15176991}, {154.0, 15177507}, {155.0, 15178019}, {156.0, 15178531}, {157.0, 15310115}, {158.0, 15441701}, {159.0, 15441959}, {160.0, 15442215}, {161.0, 15442727}, {162.0, 15443243}, {163.0, 15443755}, {164.0, 15444269}, {165.0, 15444783}, {166.0, 15444783}, {167.0, 15576367}, {168.0, 15707953}, {169.0, 15708467}, {170.0, 15708979}, {171.0, 15708981}, {172.0, 15708983}, {173.0, 15710011}, {174.0, 15710523}, {175.0, 15711037}, {176.0, 15711039}, {177.0, 15711553}, {178.0, 15843139}, {179.0, 15974213}, {180.0, 15974215}, {181.0, 15974217}, {182.0, 15974219}, {183.0, 15975755}, {184.0, 15976271}, {185.0, 15976785}, {186.0, 15977299}, {187.0, 15977301}, {188.0, 15977815}, {189.0, 15978327}, {190.0, 15978331}, {191.0, 16109917}, {192.0, 16241503}, {193.0, 16241505}, {194.0, 16242019}, {195.0, 16242535}, {196.0, 16242537}, {197.0, 16242539}, {198.0, 16243563}, {199.0, 16243567}, {200.0, 16244081}, {201.0, 16244595}, {202.0, 16244599}, {203.0, 16244601}, {204.0, 16244603}, {205.0, 16245627}, {206.0, 16245631}, {207.0, 16245633}, {208.0, 16246147}, {209.0, 16246663}, {210.0, 16377735}, {211.0, 16508811}, {212.0, 16508815}, {213.0, 16509839}, {214.0, 16509843}, {215.0, 16509845}, {216.0, 16509847}, {217.0, 16510361}, {218.0, 16510875}, {219.0, 16510879}, {220.0, 16510881}, {221.0, 16510883}, {222.0, 16511399}, {223.0, 16511911}, {224.0, 16511915}, {225.0, 16511917}, {226.0, 16511919}, {227.0, 16511923}, {228.0, 16512437}, {229.0, 16512951}, {230.0, 16512955}, {231.0, 16512957}, {232.0, 16512959}, {233.0, 16512961}, {234.0, 16512963}, {235.0, 16512967}, {236.0, 16513481}, {237.0, 16513995}, {238.0, 16513999}, {239.0, 16514001}, {240.0, 16514003}, {241.0, 16514005}, {242.0, 16514007}, {243.0, 16514011}, {244.0, 16514013}, {245.0, 16514015}, {246.0, 16514019}, {247.0, 16514021}, {248.0, 16514023}, {249.0, 16514027}, {250.0, 16514029}, {251.0, 16514031}, {252.0, 16514035}, {253.0, 16514037}, {254.0, 16514039}, {255.0, 16514043}] ("Z Scale.Marker Values[]")] -> w1012
                  tunnel: w1016 -> [w1023 w1024 w1026 w1028 w1030 w1032 w1034 w1036 w1038 w1040 w1042 w1044 w1047]
                  tunnel: [w1023 w1024 w1026 w1028 w1030 w1032 w1034 w1036 w1038 w1040 w1042 w1044 w1047] -> w1014
                  frame "System", Default {
                  }
                  frame "Fire" {
                    # "Fire"
                  }
                  frame "Gray" {
                    # "Grayscale"
                  }
                  frame "Red" {
                    # "Red"
                  }
                  frame "Green" {
                    # "Green"
                  }
                  frame "Blue" {
                    # "Blue"
                  }
                  frame "Cyan" {
                    # "Cyan"
                  }
                  frame "Magenta" {
                    # "Magenta"
                  }
                  frame "Yellow" {
                    # "Yellow"
                  }
                  frame "Red-White" {
                    # "Red-White"
                  }
                  frame "Green-White" {
                    # "Green-White"
                  }
                  frame "Blue-White" {
                    # "Blue-White"
                  }
                  frame "Glow" {
                  }
                }
                n506 = property on="Apply Color" class="Bool (strict)"(error in=w1010, "Value"=FALSE) -> ()  [unwired: 1 in, 2 out]
                n507 = property class="IntGraph (strict)"(reference=w1013, "ZScale.MarkerVals[]"=w1012, "ZScale.High Color"=u32 255, "ZScale.Maximum"=w1014) -> ()  [unwired: 1 in, 2 out]
              }
              frame "Show Cursor", Default {
                w1052 = 2.0 ("y")
                n508 = Index Array(array=w1048, index=0) -> (element=w1060:refnum<vi>)
                n509 = property class="IntGraph (strict)"(reference=w1060) -> ("Value"=w1059:sgl[][])  [unwired: 1 in, 2 out]
                n510 = Array Size(array=w1059) -> (size(s)=w1058:i32[])
                n511 = To Double Precision Float(number=w1058) -> (double precision float=w1055:dbl[])
                n512 = Index Array(array=w1055, index #1=0 ("index"), index #2=1 ("index")) -> (element #1=w1054:dbl, element #2=w1053:dbl)
                n513 = Divide(x=w1054, y=w1052) -> (x/y=w1051:dbl)
                n514 = Divide(x=w1053, y=w1052) -> (x/y=w1050:dbl)
                n515 = for {
                  tunnel: w1048 -> [w1062] mode=indexing
                  tunnel: w1051 -> [w1064]
                  tunnel: w1050 -> [w1063]
                  tunnel: w1049 -> [w1065]
                  n516 = property class="IntGraph (strict)"(reference=w1062, "Cursor.Visible"=w1065, "Cursor.Cursor X"=w1064, "Cursor.Cursor Y"=w1063) -> ()  [unwired: 1 in, 2 out]
                }
              }
              frame "Auto Scale" {
                n517 = Select(t=u8 2 ("Z Scale.Scale Fit"), s=w1069, f=u8 0) -> (s? t:f=w1066:u8)
                n518 = for {
                  tunnel: w1070 -> [w1072] mode=indexing
                  tunnel: w1066 -> [w1071]
                  n519 = property class="IntGraph (strict)"(reference=w1072, "ZScale.ScaleFit"=w1071) -> ()  [unwired: 1 in, 2 out]
                }
              }
              frame "Pan Tool", "Reset Zoom", "Zoom In", "Zoom Out" {
                n520 = case shown="\"Reset Zoom\"" w1080 {
                  tunnel: [0 ("Palette:Active Tool") 6 ("Palette:Active Tool") 7 ("Palette:Active Tool") 1 ("Palette:Active Tool") 0 ("Palette:Active Tool")] -> w1074
                  tunnel: w1073 -> [_ _ _ _ w1092]
                  frame Default {
                  }
                  frame "Zoom In" {
                  }
                  frame "Zoom Out" {
                  }
                  frame "Pan Tool" {
                  }
                  frame "Reset Zoom" {
                    n521 = property on="Reset Zoom" class="Bool (strict)"("Value"=FALSE) -> ()  [unwired: 2 in, 2 out]
                    n522 = for {
                      tunnel: w1092 -> [w1097] mode=indexing
                      tunnel: 5 ("Palette:Active Tool") -> [w1096]
                      n523 = property class="IntGraph (strict)"(reference=w1097, "ActPaletteTool"=w1096) -> ()  [unwired: 1 in, 2 out]
                    }
                  }
                }
                n524 = control-ref of="Zoom In"() -> (w1076:refnum<vi>)
                n525 = control-ref of="Zoom Out"() -> (w1078:refnum<vi>)
                n526 = control-ref of="Pan Tool"() -> (w1077:refnum<vi>)
                n527 = Build Array(w1076, w1078, w1077) -> (w1079:refnum<vi>[])
                n528 = for {
                  tunnel: w1079 -> [w1085] mode=indexing
                  tunnel: w1075 -> [w1083]
                  n529 = property class="Bool (strict)"(reference=w1085) -> (reference out=w1084:refnum<vi>, "Label.Text"=w1082:string)  [unwired: 1 in, 1 out]
                  n530 = Equal?(x=w1082, y=w1083) -> (x = y?=w1081:bool)
                  n531 = property class="Bool (strict)"(reference=w1084, "Value"=w1081) -> ()  [unwired: 1 in, 2 out]
                }
                n532 = for {
                  tunnel: w1073 -> [w1087] mode=indexing
                  tunnel: w1074 -> [w1086]
                  n533 = property class="IntGraph (strict)"(reference=w1087, "ActPaletteTool"=w1086) -> ()  [unwired: 1 in, 2 out]
                }
              }
              frame "Load File" {
                w1107 = u16 1 items=["Get Image", "Load and Read File"] ("Action")
                n534 = control-ref of="This VI"() -> (w1109:refnum<vi>)
                n535 = property on="Load File" class="Bool (strict)"("Value"=FALSE) -> ()  [unwired: 2 in, 2 out]
                n536 = call "GetDisplayClick.vi"("Display REFs In"=w1110, "Calling VI REF"=w1109) -> ("Display Index"=w1103:i32)  [unwired: 13 in]
                n537 = call "OpenDBL.vi"("Action"=w1107) -> ("Image"=w1100:sgl[], "Dimensions (Z, Y, X, t)"=w1106:i32[])  [unwired: 11 in, 2 out]
                n538 = Index Array(array=w1106, index #1=1 ("index"), index #2=2 ("index")) -> (element #1=w1099:i32, element #2=w1098:i32)
                n539 = case shown="Default" w1103 {
                  selector: w1103 -> [w1116 w1122]
                  tunnel: [w1116 w1122] -> w1102
                  tunnel: [w1112 w1117] -> w1101
                  tunnel: w1100 -> [w1115 w1121]
                  tunnel: w1099 -> [w1114 w1120]
                  tunnel: w1098 -> [w1113 w1119]
                  frame 0, 1 {
                    n540 = Reshape Array(w1115, w1114, w1113) -> (w1112:sgl[][])
                  }
                  frame Default {
                    n541 = Reshape Array(w1121, w1120, w1119) -> (w1118:sgl[][])
                    n542 = call "Rotate2DArray.vi"("Array In"=w1118) -> ("Rotated Array"=w1117:dbl[][])  [unwired: 10 in]
                  }
                }
                n543 = Index Array(array=w1110, index=w1102) -> (element=w1108:refnum<vi>)
                n544 = property class="IntGraph (strict)"(reference=w1108, "Value"=w1101) -> ()  [unwired: 1 in, 2 out]
              }
              frame "Fit Tool" {
                n545 = control-ref of="This VI"() -> (w1130:refnum<vi>)
                n546 = call "Image Aquisition Param Ctrl_AE.vi"("Action"=enum16{"READ", "WRITE"}."READ") -> ("Image Acquisition Parameters Out"=w1125:T19)  [unwired: 10 in]
                n547 = call "GetDisplayClick.vi"("Display REFs In"=w1128, "Calling VI REF"=w1130) -> ("Display Index"=w1129:i32)  [unwired: 13 in]
                n548 = Index Array(array=w1128, index=w1129) -> (element=w1127:refnum<vi>)
                n549 = property class="IntGraph (strict)"(reference=w1127) -> ("Value"=w1126:sgl[][])  [unwired: 1 in, 2 out]
                n550 = vi-ref "QuickProfile_V3.vi"() -> (w1133:refnum<vi>)
                n551 = property class="VI Interface Type 0"(reference=w1133) -> ("Path"=w1136:path)  [unwired: 1 in, 2 out]
                n552 = Unbundle By Name(w1125) -> ("Pixel Size (nm)"=w1132:dbl[])
                n553 = Index Array(array=w1132, index=0) -> (element=w1139:dbl)
                n554 = Open VI Reference(type specifier VI Refnum (for type only)=w1133, vi path=w1136, options=128) -> (vi reference=w1134:refnum<vi>)  [unwired: 3 in, 1 out]
                n555 = call-by-ref "Start Asynchronous Call"(reference=w1134, "Image IN"=w1126, "Pixel Size (nm)"=w1139) -> (reference out=w1137:refnum<vi>, error out=w1124:errorcluster)  [unwired: 15 in]
                n556 = Close Reference(reference=w1137) -> ()  [unwired: 1 in, 1 out]
                n557 = property on="Fit Tool" class="Bool (strict)"(error in=w1124, "Value"=FALSE) -> ()  [unwired: 1 in, 2 out]
              }
              frame "Smooth Tool" {
                n558 = vi-ref "SmoothTool.vi"() -> (w1144:refnum<vi>)
                n559 = property on="Smooth Tool" class="Bool (strict)"("Value"=FALSE) -> ()  [unwired: 2 in, 2 out]
                n560 = property class="VI Interface Type 1"(reference=w1144) -> ("Path"=w1146:path)  [unwired: 1 in, 2 out]
                n561 = control-ref of="This VI"() -> (w1142:refnum<vi>)
                n562 = Open VI Reference(type specifier VI Refnum (for type only)=w1144, vi path=w1146, options=128) -> (vi reference=w1145:refnum<vi>)  [unwired: 3 in, 1 out]
                n563 = call-by-ref "Start Asynchronous Call"(reference=w1145, "Calling VI REF"=w1142, "Display REFs In"=w1141) -> (reference out=w1143:refnum<vi>)  [unwired: 11 in, 1 out]
                n564 = Close Reference(reference=w1143) -> ()  [unwired: 1 in, 1 out]
              }
              frame "Merge Tool" {
                n565 = vi-ref "MergeTool - Cambridge.vi"() -> (w1152:refnum<vi>)
                n566 = property class="VI Interface Type 2"(reference=w1152) -> ("Path"=w1154:path)  [unwired: 1 in, 2 out]
                n567 = property on="Merge Tool" class="Bool (strict)"("Value"=FALSE) -> ()  [unwired: 2 in, 2 out]
                n568 = control-ref of="This VI"() -> (w1150:refnum<vi>)
                n569 = Open VI Reference(type specifier VI Refnum (for type only)=w1152, vi path=w1154, options=128) -> (vi reference=w1153:refnum<vi>)  [unwired: 3 in, 1 out]
                n570 = call-by-ref "Start Asynchronous Call"(reference=w1153, "VI Reference"=w1150, "Display References"=w1149) -> (reference out=w1151:refnum<vi>)  [unwired: 11 in, 1 out]
                n571 = Close Reference(reference=w1151) -> ()  [unwired: 1 in, 1 out]
              }
            }
          }
        }
      }
      event "Channel 1", "Channel 2", "Channel 3", "Channel 4", "Channel 5", "Channel 6": Mouse Down; "Channel 1", "Channel 2", "Channel 3", "Channel 4", "Channel 5", "Channel 6": Mouse Up {
        n572 = event-data() -> ("Type"=w1161:T30, "CtlRef"=w1158:refnum<vi>)  [unwired: 1 in, 5 out]
        n573 = Equal?(x=w1161, y=lveventtype."Mouse Down" ("Type")) -> (x = y?=w1159:bool)
        n574 = call "Graph Ref AE.vi"("Action"=enum16{"READ", "WRITE"}."READ") -> ("Graph Ref Out"=w1156:refnum<vi>[])  [unwired: 10 in]
        n575 = case shown="True" w1159 {
          tunnel: w1158 -> [w1164 w1182]
          tunnel: w1156 -> [w1163 w1181]
          frame False {
            n576 = property class="IntGraph (strict)"(reference=w1164) -> (reference out=w1168:refnum<vi>, "ActPaletteTool"=w1165:i32)  [unwired: 1 in, 1 out]
            n577 = Not Equal?(x=w1165, y=0) -> (x != y?=w1167:bool)
            n578 = case shown="False" w1167 {
              tunnel: w1168 -> [w1171 w1177]
              tunnel: w1163 -> [w1170 w1174]
              frame False {
                n579 = property class="IntGraph (strict)"(reference=w1171) -> ("Cursor.Cursor Position"=w1169:T46)  [unwired: 1 in, 2 out]
                n580 = for {
                  tunnel: w1170 -> [w1172] mode=indexing
                  tunnel: w1169 -> [w1173]
                  n581 = property class="IntGraph (strict)"(reference=w1172, "Cursor.Cursor Position"=w1173) -> ()  [unwired: 1 in, 2 out]
                }
              }
              frame True {
                n582 = property class="IntGraph (strict)"(reference=w1177) -> ("XScale.Range"=w1176:T47, "YScale.Range"=w1175:T47)  [unwired: 1 in, 2 out]
                n583 = for {
                  tunnel: w1176 -> [w1180]
                  tunnel: w1175 -> [w1179]
                  tunnel: w1174 -> [w1178] mode=indexing
                  n584 = property class="IntGraph (strict)"(reference=w1178, "XScale.Range"=w1180, "YScale.Range"=w1179) -> ()  [unwired: 1 in, 2 out]
                }
              }
            }
          }
          frame True {
            n585 = for {
              tunnel: w1181 -> [w1187] mode=indexing
              tunnel: w1182 -> [w1188]
              n586 = Equal?(x=w1187, y=w1188) -> (x = y?=w1186:bool)
              n587 = Select(t=T31 {"Left"=2431, "Top"=-324} ("Z Scale.Position"), s=w1186, f=T31 {"Left"=0, "Top"=0}) -> (s? t:f=w1183:T31)
              n588 = property class="IntGraph (strict)"(reference=w1187, "ZScale.Visible"=w1186, "ZScale.Position"=w1183) -> ()  [unwired: 1 in, 2 out]
            }
          }
        }
      }
      event "Wake Up FPGA": Value Change {
        n589 = event-data() -> ()  [unwired: 1 in, 1 out]
        n590 = flat-sequence {
          frame #0 {
            n591 = xnode "Open FPGA VI Reference"() -> ("FPGA VI Reference Out"=w1190:refnum<k20>, "error out"=w1189:errorcluster)  [unwired: 2 in]
            n592 = xnode "Close FPGA VI Reference"("FPGA VI Reference In"=w1190, "error in"=w1189) -> ()  [unwired: 1 out]
          }
          frame #1 {
            n593 = call "FPGA-7842R-Control V2.vi"("Action"=FPGA-7842R-Reference."Initialize", "Initialize"=FALSE) -> ()  [unwired: 12 in, 2 out]
          }
          frame #2 {
            n594 = One Button Dialog(message="FPGA is reinitialized!") -> ()  [unwired: 1 in, 1 out]
          }
        }
      }
      event "Sequence Cluster": Value Change {
        n595 = event-data() -> ("CtlRef"=w1197:refnum<vi>, "OldVal"=w1201:T15, "NewVal"=w1200:T15)  [unwired: 1 in]
        n596 = Not Equal?(x=w1201, y=w1200) -> (x != y?=w1199:T48)
        n597 = property class="Clust"(reference=w1197) -> ("Controls[]"=w1196:refnum<vi>[])  [unwired: 1 in, 2 out]
        n598 = Cluster To Array(cluster=w1199) -> (array=w1198:bool[])
        n599 = for {
          tunnel: w1198 -> [w1202] mode=indexing
          tunnel: w1196 -> [w1203] mode=indexing
          tunnel: [w1203] -> w1195
          stop <- w1202 stop-if-true
        }
        n600 = property class="Ctl"(reference=w1195) -> ("Label.Text"=w1194:string)  [unwired: 1 in, 2 out]
        n601 = case shown="\"DeleteSeq\"" w1194 {
          frame Default {
          }
          frame "Sequence List" {
            w1204 = enum16{"READ", "WRITE"}."WRITE" ("Action")
            n602 = property on="Sequence List" class="RadioBtnsControl (strict)"() -> ("Value"=w1209:enum32{"Seq 1", "Seq 2", "Seq 3", "Seq 4"})  [unwired: 2 in, 2 out]
            n603 = call "Seq AE.vi"("Action"=enum16{"READ", "BUILD", "WRITE", "DELETE"}."READ") -> ("Array"=w1210:T39)  [unwired: 8 in]
            n604 = Index Array(array=w1210, index=w1209) -> (element=w1208:T40)
            n605 = Unbundle By Name(w1208) -> ("Detectors Parameters Out"=w1207:T17, "Laser Parameters Out"=w1206:T18, "Image Acquisition Parameters Out"=w1205:T19)
            n606 = call "Detectors Crl_AE.vi"("Action"=w1204, "Detectors Parameters In"=w1207) -> ()  [unwired: 9 in, 1 out]
            n607 = call "LASERs_ Crl_AE.vi"("Action"=w1204, "Laser Parameters In"=w1206) -> ()  [unwired: 9 in, 1 out]
            n608 = call "Image Aquisition Param Ctrl_AE.vi"("Action"=w1204, "Image Acquisition Parameters In"=w1205) -> ()  [unwired: 9 in, 1 out]
          }
          frame "Operation Option" {
          }
          frame "AddSeq" {
            n609 = call "LASERs_ Crl_AE.vi"("Action"=enum16{"READ", "WRITE"}."READ") -> ("Laser Parameters Out"=w1216:T18)  [unwired: 10 in]
            n610 = call "Detectors Crl_AE.vi"("Action"=enum16{"READ", "WRITE"}."READ") -> ("Detectors Parameters Out"=w1217:T17)  [unwired: 10 in]
            n611 = call "Image Aquisition Param Ctrl_AE.vi"("Action"=enum16{"READ", "WRITE"}."READ") -> ("Image Acquisition Parameters Out"=w1215:T19)  [unwired: 10 in]
            n612 = Bundle("Detectors Parameters Out"=w1217, "Laser Parameters Out"=w1216, "Image Acquisition Parameters Out"=w1215) -> (w1213:T40)  [unwired: 1 in]
            n613 = property on="Sequence List" class="RadioBtnsControl (strict)"() -> ("DisabledEnum"=w1214:T25)  [unwired: 2 in, 2 out]
            n614 = case shown="\"Disabled\", \"Disabled and Grayed Out\", Default" w1214 {
              tunnel: [enum16{"READ", "BUILD", "WRITE", "DELETE"}."BUILD" ("Action") w1227] -> w1212
              frame "Disabled", "Disabled and Grayed Out", Default {
                w1222 = T25."Enabled" ("Disabled")
                n615 = property on="Sequence List" class="RadioBtnsControl (strict)"("DisabledEnum"=w1222) -> ()  [unwired: 2 in, 2 out]
                n616 = property on="Seq 1" class="Bool (strict)"("DisabledEnum"=w1222) -> ()  [unwired: 2 in, 2 out]
                n617 = property on="Seq 1" class="Bool (strict)"("Value"=TRUE) -> ()  [unwired: 2 in, 2 out]
              }
              frame "Enabled" {
                n618 = call "Seq AE.vi"("Action"=enum16{"READ", "BUILD", "WRITE", "DELETE"}."READ") -> ("Array"=w1225:T39)  [unwired: 8 in]
                n619 = Array Size(array=w1225) -> (size(s)=w1224:i32)
                n620 = case shown="1" w1224 {
                  tunnel: [enum16{"READ", "BUILD", "WRITE", "DELETE"}."READ" ("Action") enum16{"READ", "BUILD", "WRITE", "DELETE"}."WRITE" ("Action") enum16{"READ", "BUILD", "WRITE", "DELETE"}."WRITE" ("Action") enum16{"READ", "BUILD", "WRITE", "DELETE"}."WRITE" ("Action")] -> w1227
                  frame 4, Default {
                    n621 = One Button Dialog(message="No more sequence allowed!") -> ()  [unwired: 1 in, 1 out]
                  }
                  frame 1 {
                    n622 = property on="Seq 2" class="Bool (strict)"("DisabledEnum"=T25."Enabled" ("Disabled")) -> ()  [unwired: 2 in, 2 out]
                    n623 = property on="Seq 2" class="Bool (strict)"("Value"=TRUE) -> ()  [unwired: 2 in, 2 out]
                  }
                  frame 2 {
                    n624 = property on="Seq 3" class="Bool (strict)"("DisabledEnum"=T25."Enabled" ("Disabled")) -> ()  [unwired: 2 in, 2 out]
                    n625 = property on="Seq 3" class="Bool (strict)"("Value"=TRUE) -> ()  [unwired: 2 in, 2 out]
                  }
                  frame 3 {
                    n626 = property on="Seq 4" class="Bool (strict)"("DisabledEnum"=T25."Enabled" ("Disabled")) -> ()  [unwired: 2 in, 2 out]
                    n627 = property on="Seq 4" class="Bool (strict)"("Value"=TRUE) -> ()  [unwired: 2 in, 2 out]
                  }
                }
              }
            }
            n628 = call "Seq AE.vi"("Action"=w1212, "Cluster"=w1213) -> ()  [unwired: 7 in, 1 out]
          }
          frame "DeleteSeq" {
            n629 = call "Seq AE.vi"("Action"=enum16{"READ", "BUILD", "WRITE", "DELETE"}."READ") -> ("Array"=w1240:T39)  [unwired: 8 in]
            n630 = Array Size(array=w1240) -> (size(s)=w1239:i32)
            n631 = case shown="2..4" w1239 {
              selector: w1239 -> [_ _ w1245]
              frame 0, Default {
              }
              frame 1 {
                n632 = call "Seq AE.vi"("Action"=enum16{"READ", "BUILD", "WRITE", "DELETE"}."DELETE") -> ()  [unwired: 8 in, 1 out]
                n633 = property on="Sequence List" class="RadioBtnsControl (strict)"("DisabledEnum"=T25."Disabled and Grayed Out" ("Disabled")) -> ()  [unwired: 2 in, 2 out]
              }
              frame 2..4 {
                n634 = property on="Sequence List" class="RadioBtnsControl (strict)"() -> ("Value"=w1247:enum32{"Seq 1", "Seq 2", "Seq 3", "Seq 4"})  [unwired: 2 in, 2 out]
                n635 = Decrement(x=w1245) -> (x-1=w1246:i32)
                n636 = Equal?(x=w1246, y=w1247) -> (x = y?=w1248:bool)
                n637 = call "Seq AE.vi"("Action"=enum16{"READ", "BUILD", "WRITE", "DELETE"}."DELETE") -> ("Array"=w1244:T39)  [unwired: 8 in]
                n638 = case shown="4" w1245 {
                  frame 2, Default {
                    n639 = property on="Seq 2" class="Bool (strict)"("DisabledEnum"=T25."Disabled and Grayed Out" ("Disabled")) -> ()  [unwired: 2 in, 2 out]
                  }
                  frame 3 {
                    n640 = property on="Seq 3" class="Bool (strict)"("DisabledEnum"=T25."Disabled and Grayed Out" ("Disabled")) -> ()  [unwired: 2 in, 2 out]
                  }
                  frame 4 {
                    n641 = property on="Seq 4" class="Bool (strict)"("DisabledEnum"=T25."Disabled and Grayed Out" ("Disabled")) -> ()  [unwired: 2 in, 2 out]
                  }
                }
                n642 = case shown="True" w1248 {
                  tunnel: w1247 -> [_ w1260]
                  tunnel: w1244 -> [_ w1259]
                  frame False {
                  }
                  frame True {
                    w1254 = enum16{"READ", "WRITE"}."WRITE" ("Action")
                    n643 = Decrement(x=w1260) -> (x-1=w1258:enum32{"Seq 1", "Seq 2", "Seq 3", "Seq 4"})
                    n644 = Index Array(array=w1259, index=w1258) -> (element=w1253:T40)
                    n645 = property on="Sequence List" class="RadioBtnsControl (strict)"("Value"=w1258) -> ()  [unwired: 2 in, 2 out]
                    n646 = Unbundle By Name(w1253) -> ("Detectors Parameters Out"=w1257:T17, "Laser Parameters Out"=w1256:T18, "Image Acquisition Parameters Out"=w1255:T19)
                    n647 = call "Detectors Crl_AE.vi"("Action"=w1254, "Detectors Parameters In"=w1257) -> ()  [unwired: 9 in, 1 out]
                    n648 = call "LASERs_ Crl_AE.vi"("Action"=w1254, "Laser Parameters In"=w1256) -> ()  [unwired: 9 in, 1 out]
                    n649 = call "Image Aquisition Param Ctrl_AE.vi"("Action"=w1254, "Image Acquisition Parameters In"=w1255) -> ()  [unwired: 9 in, 1 out]
                  }
                }
              }
            }
          }
          frame "DeleteAllSeq" {
            n650 = call "Seq AE.vi"("Action"=enum16{"READ", "BUILD", "WRITE", "DELETE"}."READ") -> ("Array"=w1262:T39)  [unwired: 8 in]
            n651 = Array Size(array=w1262) -> (size(s)=w1261:i32)
            n652 = flat-sequence {
              tunnel: w1261 -> [w1264]
              frame #0 {
                n653 = for {
                  N: w1264 -> [_]
                  n654 = call "Seq AE.vi"("Action"=enum16{"READ", "BUILD", "WRITE", "DELETE"}."DELETE") -> ()  [unwired: 8 in, 1 out]
                }
              }
              frame #1 {
                n655 = property on="Sequence List" class="RadioBtnsControl (strict)"("DisabledEnum"=T25."Disabled and Grayed Out" ("Disabled")) -> ()  [unwired: 2 in, 2 out]
              }
            }
          }
        }
      }
      event "Exit": Value Change {
        n656 = event-data() -> ("CtlRef"=w1291:refnum<vi>, "NewVal"=w1293:bool)  [unwired: 1 in, 1 out]
        n657 = Release Notifier(notifier=w1286, force destroy? (F)=TRUE) -> ()  [unwired: 1 in, 3 out]
        n658 = property class="Bool"(reference=w1291) -> ("Label.Text"=w1290:string)  [unwired: 1 in, 2 out]
        n659 = call "SLM AE.vi"("Action"=enum16{"READ", "WRITE"}."READ") -> ("SLM Ref Out"=w1284:refnum<vi>)  [unwired: 10 in]
        n660 = call "DM_Ref_AE.vi"("Action"=enum16{"READ", "WRITE"}."READ") -> ("DM Ref Out"=w1282:refnum<vi>)  [unwired: 10 in]
        n661 = call "GateDelay AE.vi"("Action"=enum16{"READ", "WRITE"}."READ") -> ("Gate Delay Ref Out"=w1283:refnum<vi>)  [unwired: 10 in]
        n662 = Enqueue Element(queue=w1292, element=w1290) -> ()  [unwired: 2 in, 3 out]
        n663 = Build Array(w1284, w1282, w1283) -> (w1281:refnum<vi>[])
        n664 = call "Stage_position_ae.vi"("StageID"="N664", "Enum"=enum16{"WRITE", "READ", "HOME", "SAVE HOME"}."HOME") -> ("Position Out"=w1273:dbl[])  [unwired: 8 in, 1 out]
        n665 = call "Stage_position_ae.vi"("StageID"="P541", "Enum"=enum16{"WRITE", "READ", "HOME", "SAVE HOME"}."HOME") -> ("Position Out"=w1277:dbl[])  [unwired: 8 in, 1 out]
        n666 = for {
          tunnel: w1281 -> [w1298] mode=indexing
          n667 = Not A Number/Path/Refnum?(number/path/refnum=w1298) -> (NaN/Path/Refnum?=w1297:bool)
          n668 = case shown="False" w1297 {
            tunnel: w1298 -> [w1299 _]
            frame False {
              n669 = To Variant(anything=TRUE) -> (Variant=w1300:variant)
              n670 = invoke class="VI" method="Ctrl Val.Set"(reference=w1299, "Control Name"="Exit", "Value"=w1300) -> (reference out=w1303:refnum<vi>)  [unwired: 2 in, 4 out]
              n671 = Close Reference(reference=w1303) -> ()  [unwired: 1 in, 1 out]
            }
            frame True {
            }
          }
        }
        n672 = Index Array(array=w1273, index=0) -> (element=w1270:dbl)
        n673 = property on="Stages" class="Clust (strict)"() -> ("Controls[]"=w1280:refnum<vi>[])  [unwired: 2 in, 2 out]
        n674 = Index Array(array=w1277, index=0) -> (element=w1271:dbl)
        n675 = Build Array(w1271, w1270) -> (w1269:dbl[])
        n676 = for {
          tunnel: w1280 -> [w1296] mode=indexing
          n677 = property class="Ctl"(reference=w1296) -> ("Label.Text"=w1295:string)  [unwired: 1 in, 2 out]
          n678 = call "All_Stages_Aloha.vi"("Aloha"=FALSE, "Stage ID"=w1295) -> ()  [unwired: 9 in, 1 out]
        }
        n679 = call-poly <vilib>:"Write To Spreadsheet File.vi"("format (%.3f)"="%.4f", "1D data"=w1269, "file path (dialog if empty)"=path "C:/Users/ED STED/Documents/Test Control Software/Host VIs/Stages/Stage Positions/home position.csv") -> ()  [unwired: 5 in, 1 out]
      }
    }
  }
  n680 = call "Manual Controls Action Engine.vi"("Action"=enum16{"Read", "Write"}."Write", "Manual Controls In"=w31) -> ("Manual Controls Out"=w33:T21)  [unwired: 13 in]
  n681 = call "FPGA-7842R-Control V2.vi"("Action"=FPGA-7842R-Reference."Initialize", "Manual Controls"=w33, "Initialize"=FALSE) -> ("Initalized"=w15:bool)  [unwired: 11 in, 1 out]
  n682 = call "Galvo Offset AE v1.vi"("Galvo 1 Offset In"=-0.15, "Action"=enum16{"Read", "Write"}."Write") -> ("Galvo 2 Offset Out"=w1:dbl, "Galvo 1 Offset Out"=w4:dbl)
  n683 = while {
    shift-right: [w1316] -> _
    shift-left: "Idle" -> [w1317]
    tunnel: w22 -> [w1313]
    shift-right: [w1311] -> _
    shift-left: w15 -> [w1312]
    tunnel: w5 -> [w1304]
    tunnel: w4 -> [_]
    tunnel: w1 -> [_]
    stop <- w1315 stop-if-true
    n684 = call "Image Aquisition Param Ctrl_AE.vi"("Action"=enum16{"READ", "WRITE"}."READ") -> ("Image Acquisition Parameters Out"=w1310:T19)  [unwired: 10 in]
    n685 = call "Detectors Crl_AE.vi"("Action"=enum16{"READ", "WRITE"}."READ") -> ("Detectors Parameters Out"=w1308:T17)  [unwired: 10 in]
    n686 = call "Manual Controls Action Engine.vi"("Action"=enum16{"Read", "Write"}."Read") -> ("Manual Controls Out"=w1305:T21)  [unwired: 14 in]
    n687 = case shown="\"Start Waveforms\"" w1317 {
      selector: w1317 -> [_ _ _ w1339 _ _ _ _ _ _]
      tunnel: ["Exit" w1326 "Idle" ("name (unnamed)") "Arange Displays" ("name (unnamed)") "Start FPGA Acquisition" ("name (unnamed)") "Display" ("name (unnamed)") "Close Images" ("name (unnamed)") "Idle" "Stop Waveforms" ("name (unnamed)") "Start Waveforms" ("name (unnamed)")] -> w1316
      tunnel: [TRUE w1328 w1335 w1346 w1415 w1441 w1482 w1515 w1524 w1562] -> w1315
      tunnel: FALSE -> [_ w1328 w1335 w1346 w1415 w1441 w1482 w1515 w1524 w1562]
      tunnel: w1313 -> [_ w1327 _ _ _ _ _ _ _ _]
      tunnel: w1312 -> [w1322 w1325 w1336 w1341 w1412 w1439 w1480 w1513 w1516 w1563]
      tunnel: [w1321 w1325 w1336 w1340 w1412 w1435 w1480 w1512 w1516 w1563] -> w1311
      tunnel: w1310 -> [_ _ _ w1344 _ w1434 _ _ _ w1560]
      tunnel: w1308 -> [_ _ _ w1343 _ _ _ _ _ w1558]
      tunnel: w1305 -> [_ _ _ w1342 _ _ _ _ _ _]
      tunnel: w1304 -> [_ _ _ _ w1405 _ _ _ _ _]
      frame "Exit" {
        n688 = call "Graph Ref AE.vi"("Action"=enum16{"READ", "WRITE"}."READ") -> ("Graph Ref Out"=w1319:refnum<vi>[])  [unwired: 10 in]
        n689 = call "FPGA-7842R-Control V2.vi"("Action"=FPGA-7842R-Reference."Close FPGA", "Initialize"=w1322) -> ("Initalized"=w1321:bool)  [unwired: 12 in, 1 out]
        n690 = Close Reference(reference=w1319) -> ()  [unwired: 1 in, 1 out]
      }
      frame "Idle", Default {
        n691 = Dequeue Element(queue=w1327, timeout in ms (-1)=-1) -> (element=w1326:string)  [unwired: 1 in, 3 out]
      }
      frame "Close Images" {
        w1331 = u16 0 items=["Read", "Write"] ("Mode")
        w1332 = u16 0 items=["Write", "Read"] ("Mode")
        n692 = call "File Action V1.vi"("Mode"=w1331) -> ("Files Open"=w1330:bool)  [unwired: 12 in, 2 out]
        n693 = call "Image_Actions_V1.vi"("Mode"=w1332, "Action"="Trash Images") -> ()  [unwired: 12 in, 2 out]
        n694 = case shown="True" w1330 {
          frame False {
          }
          frame True {
            w1338 = u16 1 items=["Read", "Write"] ("Mode")
            n695 = call "File Action V1.vi"("Action"="Close Files", "Mode"=w1338) -> ()  [unwired: 11 in, 3 out]
          }
        }
      }
      frame "Capture", "Live", "Sequence" {
        n696 = case shown="\"Live\", Default" w1339 {
          tunnel: w1344 -> [w1362 w1383 w1399]
          tunnel: w1343 -> [w1361 w1382 w1398]
          tunnel: w1342 -> [w1352 w1373 _]
          tunnel: w1341 -> [w1351 w1372 w1389]
          tunnel: [w1351 w1372 w1389] -> w1340
          frame "Capture" {
            w1349 = u16 1 items=["Read", "Write"] ("Mode")
            w1366 = u16 0 items=["Write", "Read"] ("Mode")
            n697 = Cluster To Array(cluster=w1361) -> (array=w1359:bool[])
            n698 = Index Array(array=w1359, index=4) -> (element=w1356:bool)
            n699 = Boolean To (0,1)(Boolean=w1359) -> (0, 1=w1360:i16[])
            n700 = Add Array Elements(numeric array=w1360) -> (sum=w1357:i16)
            n701 = To Long Integer(number=w1357) -> (32bit integer=w1354:i32)
            n702 = Unbundle By Name(w1362) -> ("Image Format"=w1363:u16)
            n703 = Select(t=1, s=w1356, f=w1354) -> (s? t:f=w1353:i32)
            n704 = call "File Action V1.vi"("Action"="Open Files", "Mode"=w1349, "Image Acquisition Parameters"=w1362, "Manual Controls In"=w1352, "File Path IN"="Save File Path", "Number of Channels"=w1353) -> ("File Path OUT"=w1347:path)  [unwired: 7 in, 2 out]
            n705 = local write "Save File Path"(w1347) -> ()
            n706 = To Long Integer(number=w1363) -> (32bit integer=w1365:i32)
            n707 = Bundle(w1365, w1365) -> (w1364:cluster{i32, i32})  [unwired: 1 in]
            n708 = call "Image_Actions_V1.vi"("Image Size (Pixels)"=w1364, "Mode"=w1366, "Number of Channels"=w1353, "Action"="Create Images") -> ()  [unwired: 10 in, 2 out]
          }
          frame "Sequence" {
            w1370 = u16 1 items=["Read", "Write"] ("Mode")
            w1387 = u16 0 items=["Write", "Read"] ("Mode")
            n709 = local read "Save File Path"() -> (w1369:path)
            n710 = Cluster To Array(cluster=w1382) -> (array=w1380:bool[])
            n711 = Index Array(array=w1380, index=4) -> (element=w1377:bool)
            n712 = Boolean To (0,1)(Boolean=w1380) -> (0, 1=w1381:i16[])
            n713 = Add Array Elements(numeric array=w1381) -> (sum=w1378:i16)
            n714 = To Long Integer(number=w1378) -> (32bit integer=w1375:i32)
            n715 = Unbundle By Name(w1383) -> ("Image Format"=w1384:u16)
            n716 = Select(t=1, s=w1377, f=w1375) -> (s? t:f=w1374:i32)
            n717 = call "File Action V1.vi"("Action"="Open Files", "Mode"=w1370, "Image Acquisition Parameters"=w1383, "Manual Controls In"=w1373, "File Path IN"=w1369, "Number of Channels"=w1374) -> ("File Path OUT"=w1368:path)  [unwired: 7 in, 2 out]
            n718 = local write "Save File Path"(w1368) -> ()
            n719 = To Long Integer(number=w1384) -> (32bit integer=w1386:i32)
            n720 = Bundle(w1386, w1386) -> (w1385:cluster{i32, i32})  [unwired: 1 in]
            n721 = call "Image_Actions_V1.vi"("Image Size (Pixels)"=w1385, "Mode"=w1387, "Number of Channels"=w1374, "Action"="Create Images") -> ()  [unwired: 10 in, 2 out]
          }
          frame "Live", Default {
            w1403 = u16 0 items=["Write", "Read"] ("Mode")
            n722 = Cluster To Array(cluster=w1398) -> (array=w1396:bool[])
            n723 = Index Array(array=w1396, index=4) -> (element=w1393:bool)
            n724 = Boolean To (0,1)(Boolean=w1396) -> (0, 1=w1397:i16[])
            n725 = Add Array Elements(numeric array=w1397) -> (sum=w1394:i16)
            n726 = To Long Integer(number=w1394) -> (32bit integer=w1391:i32)
            n727 = Unbundle By Name(w1399) -> ("Image Format"=w1400:u16)
            n728 = Select(t=1, s=w1393, f=w1391) -> (s? t:f=w1390:i32)
            n729 = To Long Integer(number=w1400) -> (32bit integer=w1402:i32)
            n730 = Bundle(w1402, w1402) -> (w1401:cluster{i32, i32})  [unwired: 1 in]
            n731 = call "Image_Actions_V1.vi"("Image Size (Pixels)"=w1401, "Mode"=w1403, "Number of Channels"=w1390, "Action"="Create Images") -> ()  [unwired: 10 in, 2 out]
          }
        }
      }
      frame "Arange Displays" {
        w1410 = u16 1 items=["Write", "Read"] ("Mode")
        w1413 = u16 1 items=["Read", "Write"] ("Action")
        n732 = call "Image_Actions_V1.vi"("Mode"=w1410) -> ("Image REFs OUT"=w1411:T49[])  [unwired: 13 in, 1 out]
        n733 = call "Graph Ref AE.vi"("Action"=enum16{"READ", "WRITE"}."READ", "Graph Ref In"=w1405) -> ("Graph Ref Out"=w1407:refnum<vi>[])  [unwired: 9 in]
        n734 = Array Size(array=w1411) -> (size(s)=w1409:i32)
        n735 = call "Arange_Displays_V2.vi"("Display References"=w1407, "Action"=w1413, "Number of Channels"=w1409, "Aspect Ratio (h/w)"=1.0) -> ("Number of Channels OUT"=w1408:i32)  [unwired: 11 in]
        n736 = for {
          N: w1408 -> [_]
          tunnel: w1407 -> [w1417] mode=indexing
          tunnel: [w1420] -> _ mode=indexing
          i -> [w1418]
          n737 = property class="IntGraph (strict)"(reference=w1417) -> ("Label.Text"=w1422:string)  [unwired: 1 in, 2 out]
          n738 = Equal To 0?(x=w1418) -> (x = 0?=w1419:bool)
          n739 = case shown="True" w1419 {
            tunnel: w1417 -> [_ w1423]
            frame False {
            }
            frame True {
              n740 = property class="IntGraph (strict)"(reference=w1423, "ZScale.Visible"=TRUE ("Z Scale.Visible"), "ZScale.Position"=T31 {"Left"=2431, "Top"=-320} ("Z Scale.Position")) -> ()  [unwired: 1 in, 2 out]
            }
          }
          n741 = To Unsigned Word Integer(number=w1418) -> (unsigned 16bit integer=w1421:u16)
          n742 = Bundle("Label.Text"=w1422, w1421) -> (w1420:cluster{"Label.Text":string, u16})  [unwired: 1 in]
        }
        "Graph Ref Out" <- w1405
      }
      frame "Start Waveforms" {
        n743 = call "Galvo Offset AE v1.vi"("Action"=enum16{"Read", "Write"}."Read") -> ("Galvo 1 Offset Out"=w1426:dbl)  [unwired: 1 in, 1 out]
        n744 = Unbundle By Name("Laser Controls 2") -> ("Laser On Time (Ticks)"=w1429:i8, "Laser Delay (Ticks)"=w1428:i8)
        n745 = call "Initialize Waveforms V4.vi"("Image Acquisition Parameters"=w1434, "Yale Galvo 1 Offset (V)"=w1426) -> ("Waveform Data to FPGA"=w1440:T50)  [unwired: 13 in]
        n746 = Unbundle By Name(w1434) -> ("Scan Type"=w1433:enum16{"Sample Scanning", "Beam Scanning"})
        n747 = call "FPGA-7842R-Control V2.vi"("Waveform Data"=w1440, "Action"=FPGA-7842R-Reference."Start Waveforms", "Laser On Time (Ticks)"=w1429, "Image Acquisition Parameters"=w1434, "Initialize"=w1439, "Laser Delay (Ticks)"=w1428) -> ("Initalized"=w1436:bool)  [unwired: 8 in, 1 out]
        n748 = Equal?(x=w1433, y=enum16{"Sample Scanning", "Beam Scanning"}."Sample Scanning" ("Scan Type")) -> (x = y?=w1431:bool)
        n749 = case shown="True" w1431 {
          tunnel: w1436 -> [w1442 w1447]
          tunnel: [w1442 w1446] -> w1435
          frame False {
          }
          frame True {
            n750 = call "Scan Parameters Action Engine.vi"("Action"=enum16{"Read", "Write"}."Read") -> ("Scan Parameters OUT"=w1444:T20)  [unwired: 14 in]
            n751 = Unbundle By Name(w1444) -> ("Unused_Axis_I16"=w1443:i16)
            n752 = call "FPGA-7842R-Control V2.vi"("Action"=FPGA-7842R-Reference."Unused Axis I16", "Initialize"=w1447, "Unused Axis Offset (I16)"=w1443) -> ("Initalized"=w1446:bool)  [unwired: 11 in, 1 out]
          }
        }
      }
      frame "Display" {
        w1475 = u16 1 items=["Write", "Read"] ("Mode")
        n753 = call "Image_Actions_V1.vi"("Mode"=w1475) -> ("Image REFs OUT"=w1477:T49[])  [unwired: 13 in, 1 out]
        n754 = Array Size(array=w1477) -> (size(s)=w1473:i32)
        n755 = Decrement(x=w1473) -> (x-1=w1472:i32)
        n756 = for {
          N: 6 -> [_]
          tunnel: w1472 -> [w1510]
          tunnel: [w1508] -> w1476 mode=indexing
          i -> [w1509]
          n757 = Greater Or Equal?(x=w1510, y=w1509) -> (x >= y?=w1508:bool)
        }
        n758 = Obtain Notifier(name (unnamed)="Running", notification data type=FALSE) -> (notifier out=w1449:refnum<notifier>)  [unwired: 2 in, 2 out]
        n759 = Index Array(array=w1476, index #1=1 ("index"), index #2=2 ("index"), index #3=3 ("index"), index #4=4 ("index"), index #5=5 ("index")) -> (element #1=w1461:bool, element #2=w1460:bool, element #3=w1459:bool, element #4=w1458:bool, element #5=w1457:bool)
        n760 = Index Array(array=w1477, index #1=0 ("index"), index #2=1 ("index"), index #3=2 ("index"), index #4=3 ("index"), index #5=4 ("index"), index #6=5 ("index")) -> (element #1=w1456:T49, element #2=w1455:T49, element #3=w1454:T49, element #4=w1453:T49, element #5=w1452:T49, element #6=w1451:T49)
        n761 = while {
          tunnel: w1461 -> [w1497]
          tunnel: w1460 -> [w1496]
          tunnel: w1459 -> [w1492]
          tunnel: w1458 -> [w1489]
          tunnel: w1457 -> [w1488]
          tunnel: w1456 -> [w1495]
          tunnel: w1455 -> [w1494]
          tunnel: w1454 -> [w1493]
          tunnel: w1453 -> [w1491]
          tunnel: w1452 -> [w1487]
          tunnel: w1451 -> [w1490]
          tunnel: w1449 -> [w1484]
          stop <- w1485 stop-if-true
          n762 = Get Notifier Status(notifier=w1484) -> (current notification=w1485:bool)  [unwired: 1 in, 4 out]
          n763 = case shown="True" w1497 {
            tunnel: w1494 -> [_ w1507]
            frame False {
            }
            frame True {
              n764 = call "IMAQ ImageToArray"("Image"=w1507) -> ("Image Pixels (Float)"=→"Channel 2":sgl[][])  [unwired: 3 in, 4 out]
            }
          }
          n765 = case shown="False" w1496 {
            tunnel: w1493 -> [_ w1505]
            frame False {
            }
            frame True {
              n766 = call "IMAQ ImageToArray"("Image"=w1505) -> ("Image Pixels (Float)"=→"Channel 3":sgl[][])  [unwired: 3 in, 4 out]
            }
          }
          n767 = call "IMAQ ImageToArray"("Image"=w1495) -> ("Image Pixels (Float)"=→"Channel 1":sgl[][])  [unwired: 3 in, 4 out]
          n768 = case shown="False" w1492 {
            tunnel: w1491 -> [_ w1503]
            frame False {
            }
            frame True {
              n769 = call "IMAQ ImageToArray"("Image"=w1503) -> ("Image Pixels (Float)"=→"Channel 4":sgl[][])  [unwired: 3 in, 4 out]
            }
          }
          n770 = case shown="False" w1489 {
            tunnel: w1487 -> [_ w1501]
            frame False {
            }
            frame True {
              n771 = call "IMAQ ImageToArray"("Image"=w1501) -> ("Image Pixels (Float)"=→"Channel 5":sgl[][])  [unwired: 3 in, 4 out]
            }
          }
          n772 = case shown="False" w1488 {
            tunnel: w1490 -> [_ w1499]
            frame False {
            }
            frame True {
              n773 = call "IMAQ ImageToArray"("Image"=w1499) -> ("Image Pixels (Float)"=→"Channel 6":sgl[][])  [unwired: 3 in, 4 out]
            }
          }
          n774 = Wait (ms)(milliseconds to wait=u32 100) -> ()  [unwired: 1 out]
        }
      }
      frame "Stop Waveforms" {
        n775 = call "FPGA-7842R-Control V2.vi"("Action"=FPGA-7842R-Reference."Stop Waveforms", "Initialize"=w1513) -> ("Initalized"=w1512:bool)  [unwired: 12 in, 1 out]
      }
      frame "Stop Acquisition" {
        n776 = call "FPGA-7842R-Control V2.vi"("Action"=FPGA-7842R-Reference."Laser Control", "Laser Controls"=T18 {"STED Power (V)"=0.0, "STED"=FALSE, "650 nm"=FALSE, "590 nm"=FALSE, "485 nm"=FALSE, "Manual Control"=FALSE} ("Laser Controls 2"), "Initialize"=TRUE) -> ()  [unwired: 11 in, 2 out]
        n777 = call "AO AE.vi"("Action"=enum16{"READ", "WRITE"}."READ") -> ("Z Comp. Output"=w1518:T1)  [unwired: 8 in, 2 out]
        n778 = Unbundle By Name(w1518) -> ("Enable"=w1517:bool)
        n779 = case shown="True" w1517 {
          frame False {
          }
          frame True {
            n780 = call "Image Aquisition Param Ctrl_AE.vi"("Action"=enum16{"READ", "WRITE"}."READ") -> ("Image Acquisition Parameters Out"=w1528:T19)  [unwired: 10 in]
            n781 = Unbundle By Name(w1528) -> ("Scan Mode"=w1527:enum16{"XY", "XZ", "YZ", "XYZ"})
            n782 = Equal?(x=w1527, y=enum16{"XY", "XZ", "YZ", "XYZ"}."XYZ") -> (x = y?=w1525:bool)
            n783 = case shown="False" w1525 {
              frame False {
              }
              frame True {
                w1532 = 1 ("disabled index (col)")
                w1534 = 0 ("disabled index (col)")
                n784 = call "AO AE.vi"("Action"=enum16{"READ", "WRITE"}."READ") -> ("Mirror Modes Out"=w1536:T38, "DM Value Output"=w1539:dbl[][], "Z Comp. Output"=w1550:T1)  [unwired: 8 in]
                n785 = call "Mirror_Mode_DUAL_AE.vi"("Action"=Standard_Action."Write", "Mirror Modes In"=w1536) -> ()  [unwired: 13 in, 1 out]
                n786 = call "Deform_Mirror_DUAL_AE_V2.vi"("Action"=Standard_Action."Read") -> ("Refnum Out"=w1544:refnum<k7>, "Multi Map Data Out"=w1542:i32[])  [unwired: 10 in, 3 out]
                n787 = Index Array(array=w1539, index (col)=w1534) -> (element=w1535:dbl[])  [unwired: 1 in]
                n788 = Unbundle By Name(w1550) -> ("Origin (um)"=w1553:dbl)
                n789 = call "Voltage vs Signal_Data Engine_V1.vi"("Control Signal In (-1~1)"=w1535, "DM #"=w1534) -> ("Voltage Out (0~Max. Vol.)"=w1533:dbl[])  [unwired: 1 in, 1 out]
                n790 = control-ref of="Abort AllStage"() -> (w1546:refnum<vi>)
                n791 = call "WriteDM_V2.vi"("reference in"=w1544, "nDevId"=0, "MultiDM  Mapping"=w1542, "Voltage Array in"=w1533) -> ("reference out"=w1543:refnum<k7>)  [unwired: 2 in, 1 out]
                n792 = Build Array(w1553) -> (w1552:dbl[])
                n793 = Bundle By Name(cluster=w1550, "Enable"=FALSE) -> (w1548:T1)
                n794 = Index Array(array=w1539, index (col)=w1532) -> (element=w1531:dbl[])  [unwired: 1 in]
                n795 = call "AE_AllStages_Action V2.vi"("Velocity"=10000.0, "Abort"=w1546, "Positions"=w1552, "Axis"=bool[] [TRUE], "Stage ID"="P841", "Action"=StageStates."MOVE") -> ()  [unwired: 3 in, 3 out]
                n796 = call "Voltage vs Signal_Data Engine_V1.vi"("Control Signal In (-1~1)"=w1531, "DM #"=w1532) -> ("Voltage Out (0~Max. Vol.)"=w1530:dbl[])  [unwired: 1 in, 1 out]
                n797 = call "WriteDM_V2.vi"("reference in"=w1543, "nDevId"=1, "MultiDM  Mapping"=w1542, "Voltage Array in"=w1530) -> ()  [unwired: 2 in, 2 out]
                n798 = call "AO AE.vi"("Mirror Modes In"=w1536, "DM Value Input"=w1539, "Z Comp. Input"=w1548, "Action"=enum16{"READ", "WRITE"}."WRITE") -> ()  [unwired: 5 in, 3 out]
                n799 = call "Pixel Value (-1 to 1) DUAL AE.vi"("Action"=Standard_Action."Write", "Pixel Value (-1 to 1)"=w1539) -> ()  [unwired: 13 in, 1 out]
              }
            }
          }
        }
      }
      frame "Start FPGA Acquisition" {
        n800 = Unbundle By Name(w1560) -> ("Scan Mode"=w1559:enum16{"XY", "XZ", "YZ", "XYZ"})
        n801 = case shown="\"XZ\", Default" w1559 {
          tunnel: w1560 -> [_ w1571]
          tunnel: w1558 -> [_ w1570]
          frame "YZ" {
            n802 = vi-ref "FPGA Sample Scanning V1.vi"() -> (w1566:refnum<vi>)
            n803 = property class="VI Interface Type 3"(reference=w1566) -> ("Path"=w1564:path)  [unwired: 1 in, 2 out]
            n804 = Open VI Reference(type specifier VI Refnum (for type only)=w1566, vi path=w1564, options=128) -> (vi reference=w1567:refnum<vi>)  [unwired: 3 in, 1 out]
            n805 = call-by-ref "Start Asynchronous Call"(reference=w1567) -> (reference out=w1568:refnum<vi>)  [unwired: 4 in, 1 out]
            n806 = Close Reference(reference=w1568) -> ()  [unwired: 1 in, 1 out]
          }
          frame "XZ", Default {
            n807 = vi-ref "FPGA Beam Scanning V2.vi"() -> (w1573:refnum<vi>)
            n808 = property class="VI Interface Type 4"(reference=w1573) -> ("Path"=w1574:path)  [unwired: 1 in, 2 out]
            n809 = Open VI Reference(type specifier VI Refnum (for type only)=w1573, vi path=w1574, options=128) -> (vi reference=w1572:refnum<vi>)  [unwired: 3 in, 1 out]
            n810 = call-by-ref "Start Asynchronous Call"(reference=w1572, "Detectors"=w1570, "Image Acquisition Parameters"=w1571) -> (reference out=w1569:refnum<vi>)  [unwired: 3 in, 1 out]
            n811 = Close Reference(reference=w1569) -> ()  [unwired: 1 in, 1 out]
          }
        }
      }
    }
  }
